vi "上下管柱装配.vi"() -> ()   [LabVIEW 2020]
uses:
  Global_Variable/A131258.vi
  Global_Variable/Global.vi
  Database/Global1.vi
  <vilib>/addons/database/NI_Database_API.lvlib
  <vilib>/addons/database/Connection.llb/Conn Execute.vi
  <vilib>/addons/database/Recordset.llb/Rec Fetch Recordset Data (R).vi
  <vilib>/addons/database/Connection.llb/DB Tools Open Connec (String).vi
panel:
  in  "STEP":string
  out "左压装下限":dbl format="%#.2f"
  out "左压装上限":dbl format="%#.2f"
  out "左下限2":dbl format="%#.2f"
  out "左上限2":dbl format="%#.2f"
  out "左下限1":dbl format="%#.2f"
  out "左上限1":dbl format="%#.2f"
  out "压装最大位移(mm)":dbl
  out "判定结果":bool
  out "位移区间最大压力(KN)":dbl
  out "位移区间最小压力(KN)":dbl
  out "标尺改变":refnum<user-event>
  out "试验项":refnum<user-event>
  out "上序结果":string
  out "RIGHTMIN压力":string
  out "RIGHTMAX压力":string
  out "RIGHT位移":string
  out "LEFTMIN压力":string
  out "LEFTMAX压力":string
  out "LEFT位移":string
  out "RESULT":string
  out "PRODUCTID":string
  out "USERID":string
  out "上管柱码":string
  out "前序deviceID":string
  out "deviceID":string
  out "CODE_ID":string
  in  "判定结果 3":bool[][](array[boolean])=[[TRUE]]
  out "选项卡控件 2":enum32{"左工位压装曲线", "右工位压装曲线 ", "参数查看"}(tab)
  out "左工位曲线":cluster{dbl[], dbl[]}[](graph)
  out "右位移下限":dbl format="%#.2f"
  out "右位移上限":dbl format="%#.2f"
  out "右下限2":dbl format="%#.2f"
  out "右上限2":dbl format="%#.2f"
  out "右下限1":dbl format="%#.2f"
  out "右上限1":dbl format="%#.2f"
  out "压装最大位移(mm) 2":dbl
  out "判定结果 2":bool
  out "右工位曲线":cluster{dbl[], dbl[]}[](graph)
  out "位移区间最大压力(KN) 2":dbl
  out "位移区间最小压力(KN) 2":dbl
  in  "删除":bool
  in  "确定":bool
  in  "添加":bool
  in  "退出":bool
  in  "更新":bool
  in  "产品型号":string(combo)
  in  "选项卡控件 3":enum32{"左工位参数", "右工位参数", "产品管理", "用户管理"}(tab)
  in  "左工位坐标轴参数":string[][](table)=[["mm"], ["mm/s"]]
  in  "左工位判定框参数":string[][](table)=[["mm"], ["mm/s"]]
  in  "左工位结果判定参数":string[][](table)=[["mm"], ["mm/s"]]
  in  "右工位结果判定参数":string[][](table)=[["mm"], ["mm/s"]]
  in  "右工位判定框参数":string[][](table)=[["mm"], ["mm/s"]]
  in  "右工位坐标轴参数":string[][](table)=[["mm"], ["mm/s"]]
  in  "确定按钮":bool
  # "上限"
  # "下限"
  # "上序状态"
  # "上限"
  # "下限"
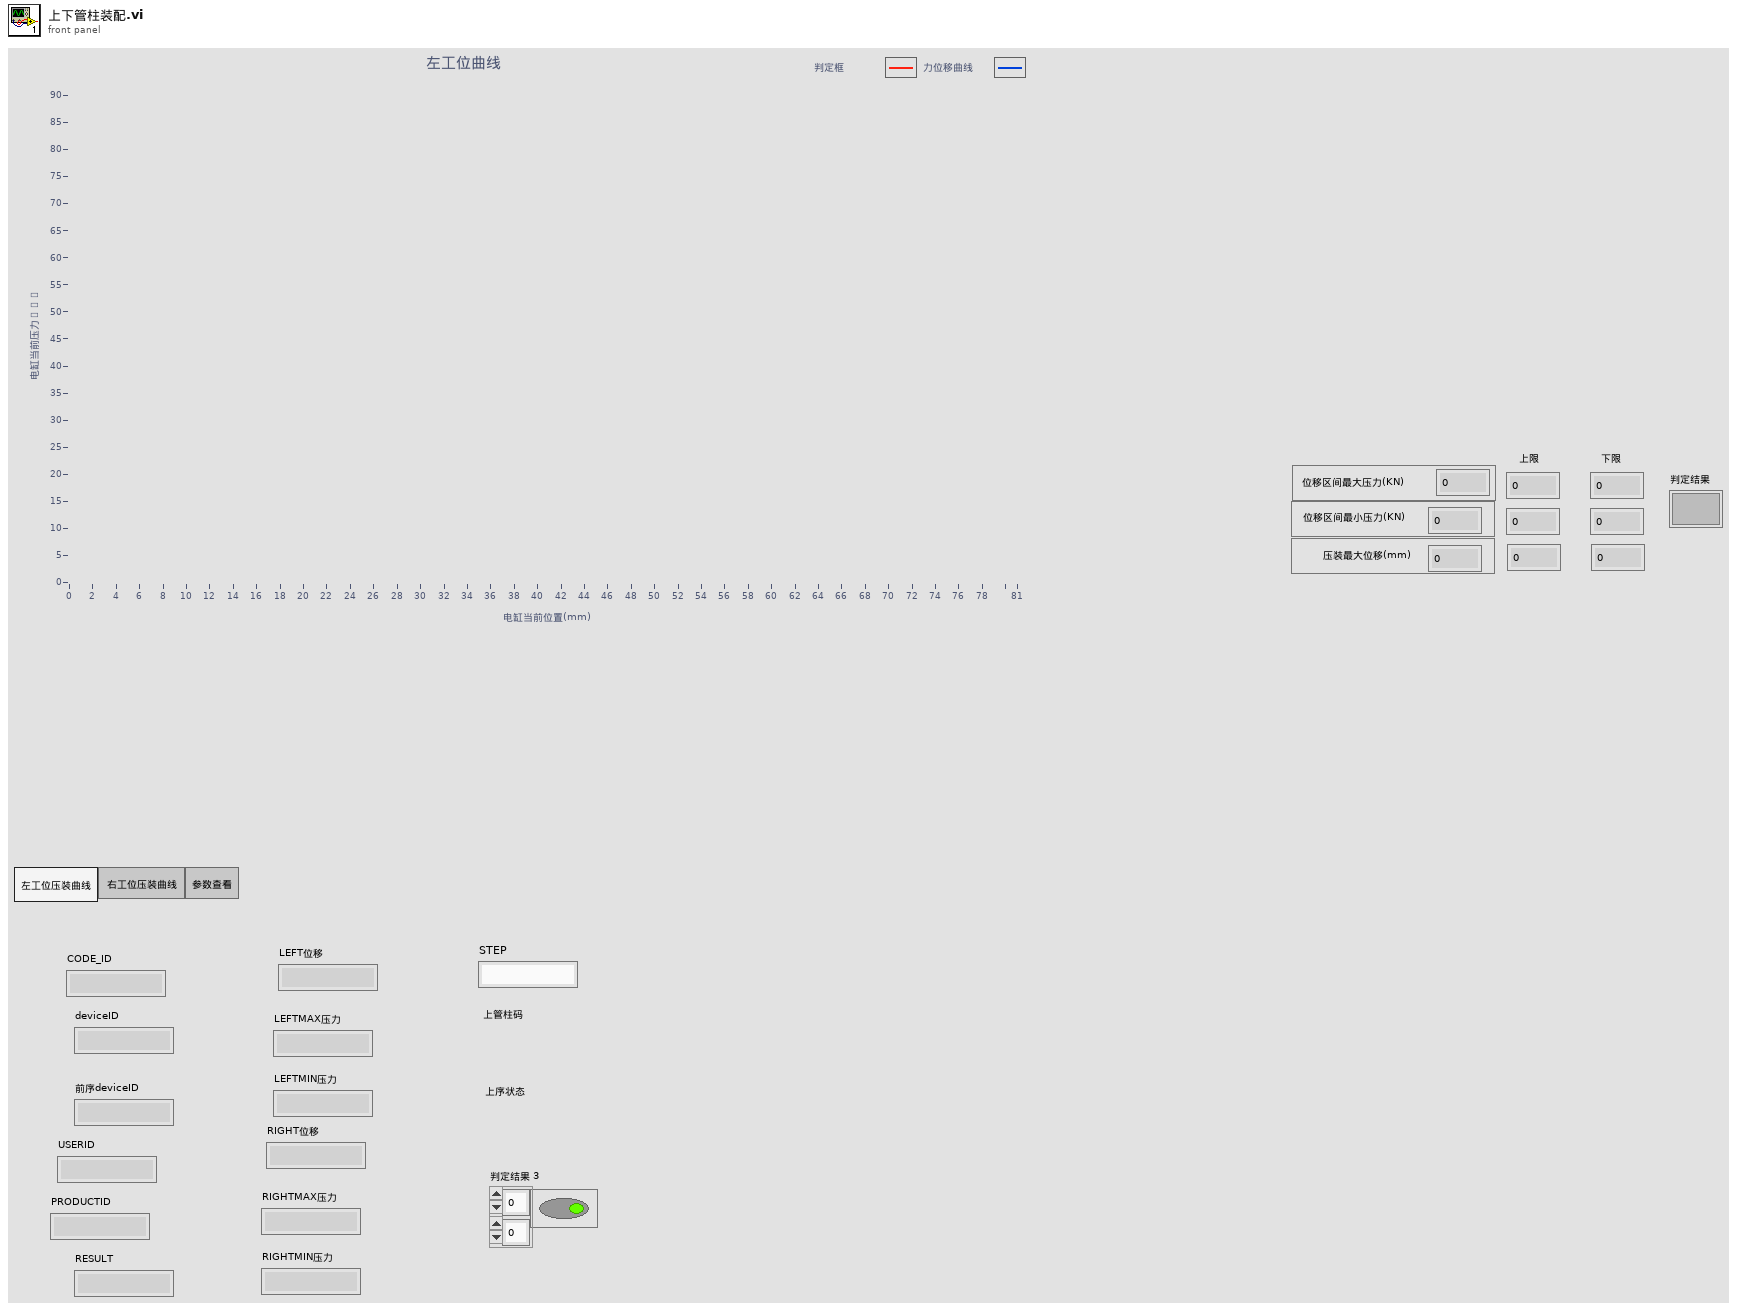
[diagram p1: front panel]
types:
  T1 = cluster{"X ":cluster{"单位":string, "下限":dbl, "上限":dbl}, "Y":cluster{"单位":string, "下限":dbl, "上限":dbl}}
  T2 = cluster{"左工位最大压力 ":cluster{"单位":string, "下限":dbl, "上限":dbl}, "左工位最小压力":cluster{"单位":string, "下限":dbl, "上限":dbl}, "左工位最终压装位移":cluster{"单位":string, "下限":dbl, "上限":dbl}}
  T3 = cluster{"右工位最大压力 ":cluster{"单位":string, "下限":dbl, "上限":dbl}, "右工位最小压力":cluster{"单位":string, "下限":dbl, "上限":dbl}, "右工位最最终位移":cluster{"单位":string, "下限":dbl, "上限":dbl}}
  T4 = cluster{i64, i64, "table":string, "压装最大位移(mm) 2":dbl, "右位移下限":dbl, "右位移上限":dbl, "table":string, "RIGHT位移":string}
  T5 = cluster{i64, i64, "table":string, "位移区间最大压力(KN) 2":dbl, "右下限1":dbl, "右上限1":dbl, "table":string, "RIGHTMAX压力":string}
  T6 = cluster{i64, i64, "table":string, "位移区间最小压力(KN) 2":dbl, "右下限2":dbl, "右上限2":dbl, "table":string, "RIGHTMIN压力":string}
  T7 = cluster{i64, i64, "table":string, "位移区间最小压力(KN) 2":dbl, "右下限2":dbl, "右上限2":dbl, "table":string, "RIGHTMIN压力":string}[]
  T8 = typedef "NI_Database_API.lvlib/Conn ObjectReference.ctl" = refnum<k1>
  T9 = cluster{i64, i64, "位移区间最小压力(KN) 2":dbl, "右下限2":dbl, "右上限2":dbl, "table":string, "RIGHTMIN压力":string}
  T10 = cluster{i64, i64, i64, "RESULT":string, "result string":string}
  T11 = cluster{i64, i64, i64, "RESULT":string, "result string":string}[]
  T12 = typedef "NI_Database_API.lvlib/Rec ObjectReference.ctl" = refnum<k1>
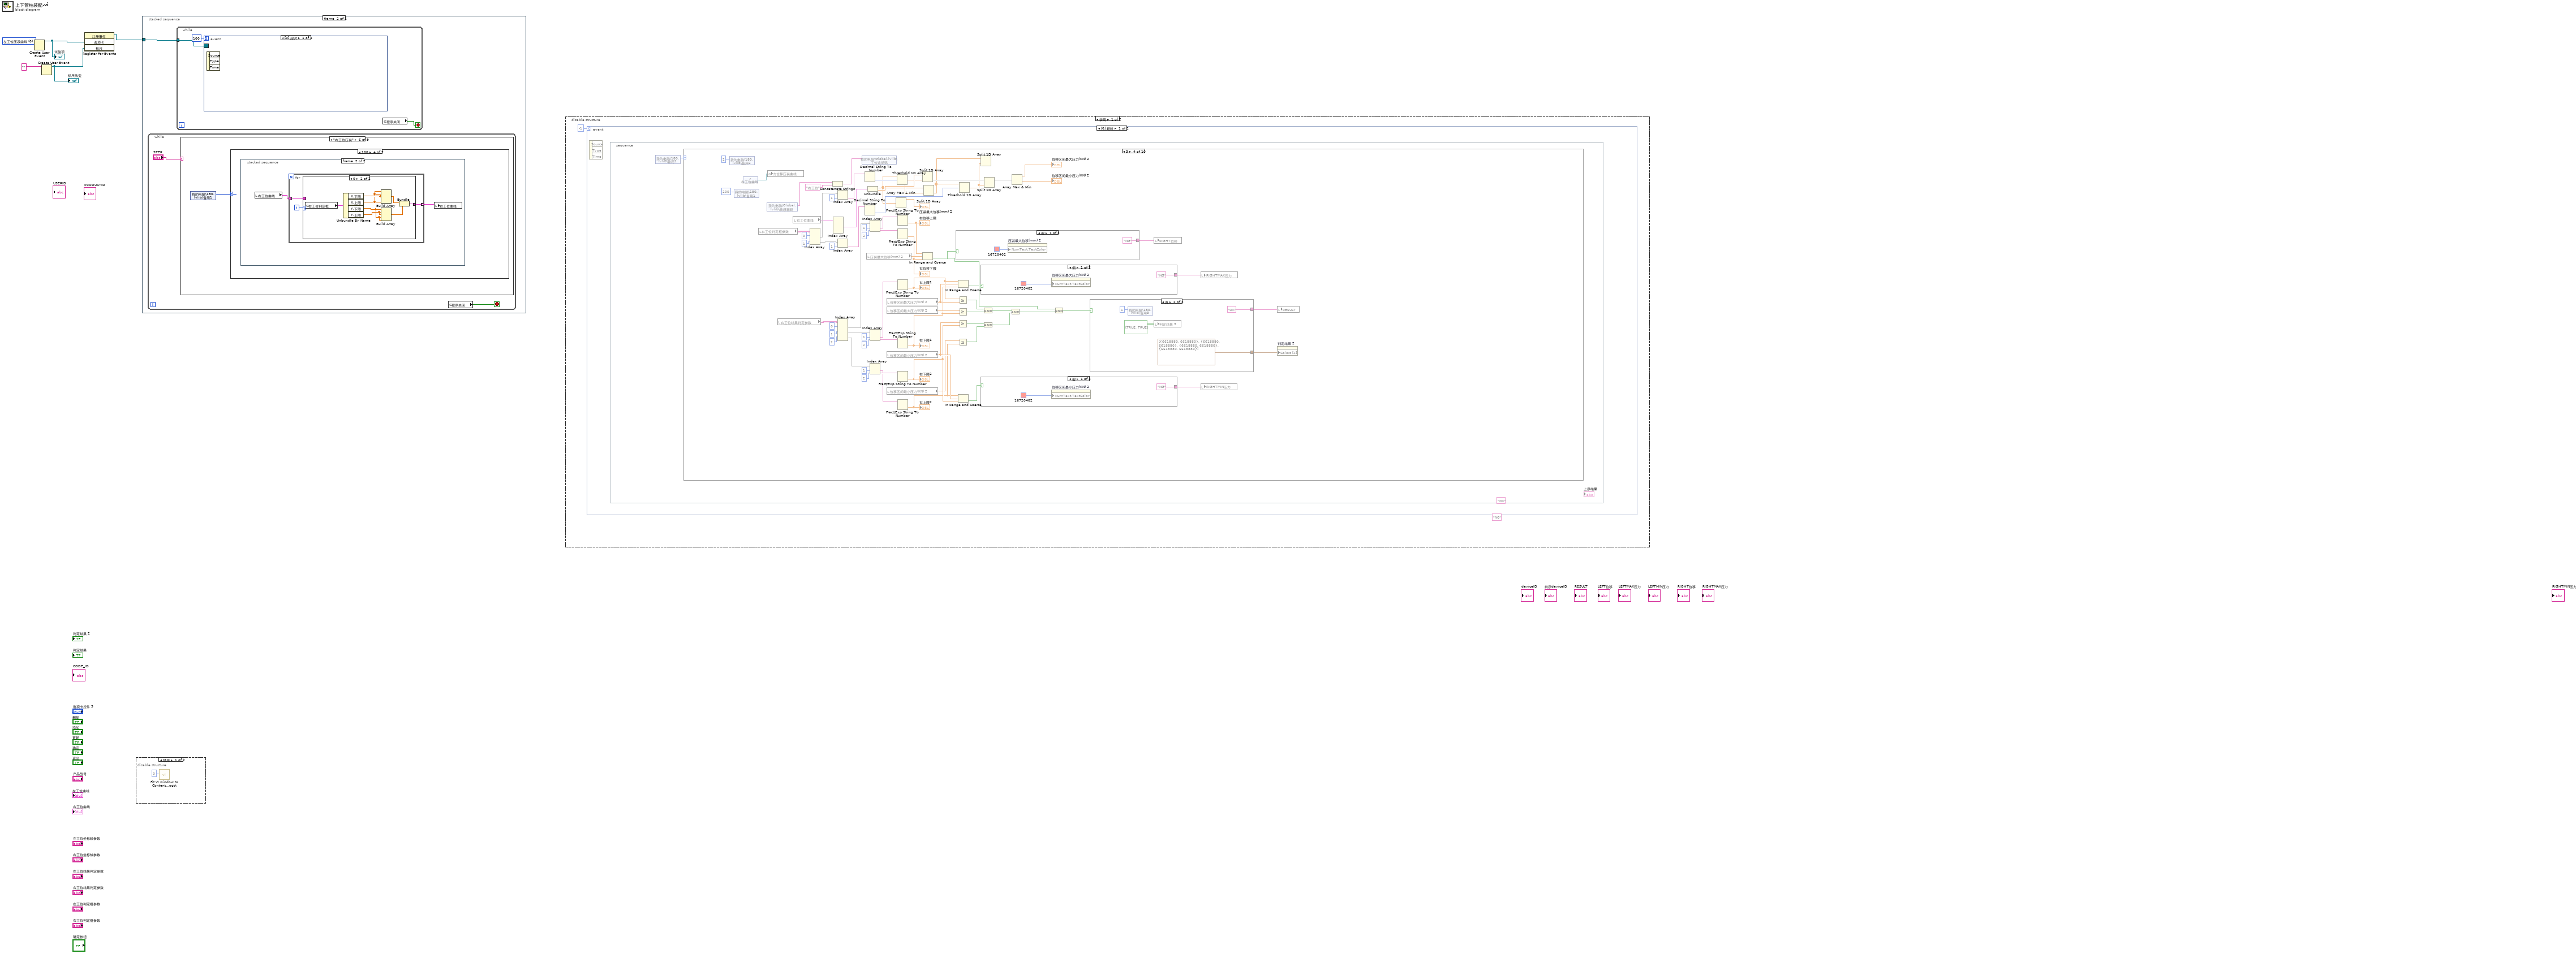
[diagram p0: block diagram]
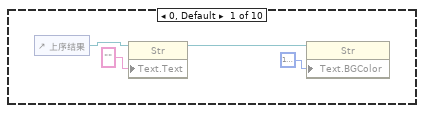
[diagram p2: hidden frame]
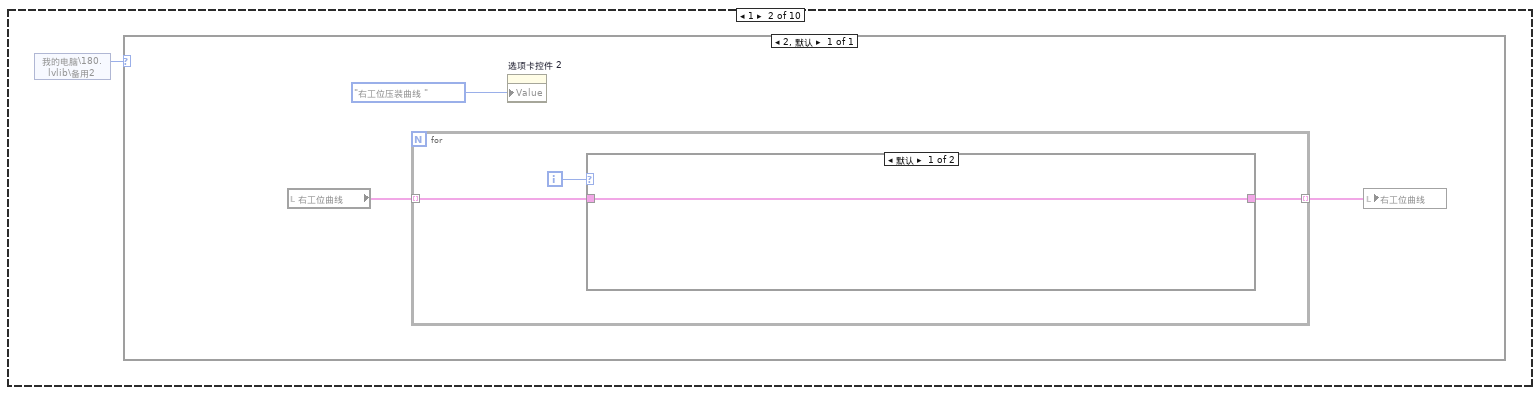
[diagram p3: hidden frame]
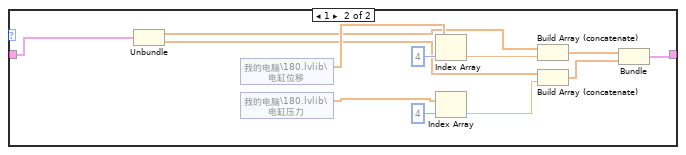
[diagram p4: hidden frame]
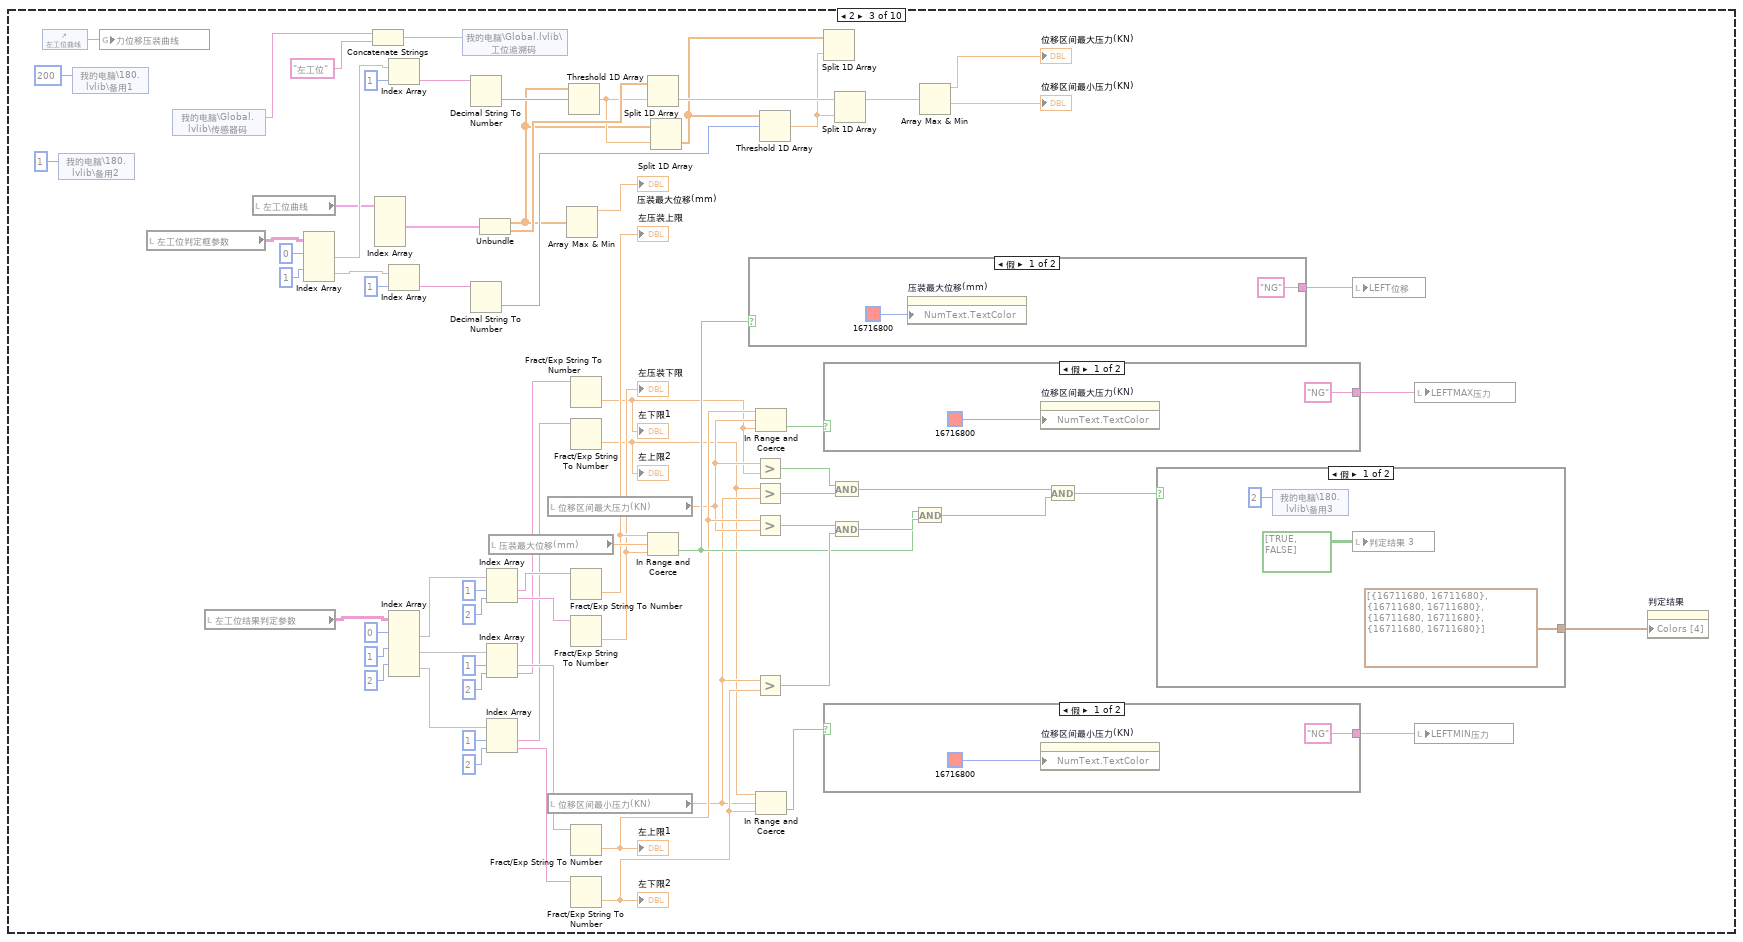
[diagram p5: hidden frame]
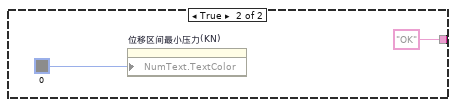
[diagram p6: hidden frame]
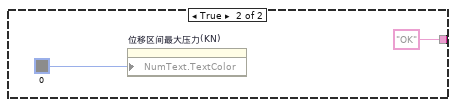
[diagram p7: hidden frame]
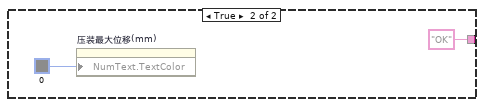
[diagram p8: hidden frame]
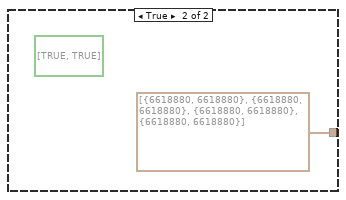
[diagram p9: hidden frame]
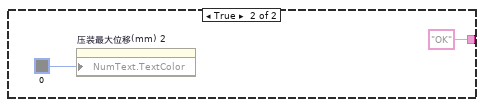
[diagram p10: hidden frame]
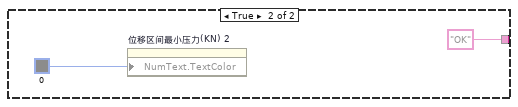
[diagram p11: hidden frame]
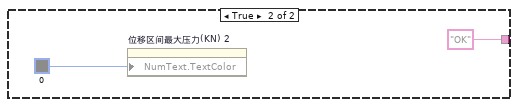
[diagram p12: hidden frame]
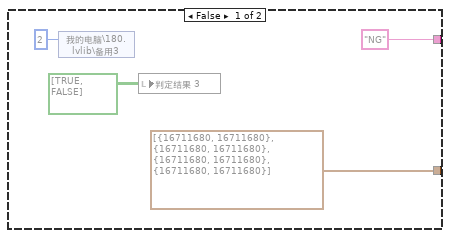
[diagram p13: hidden frame]
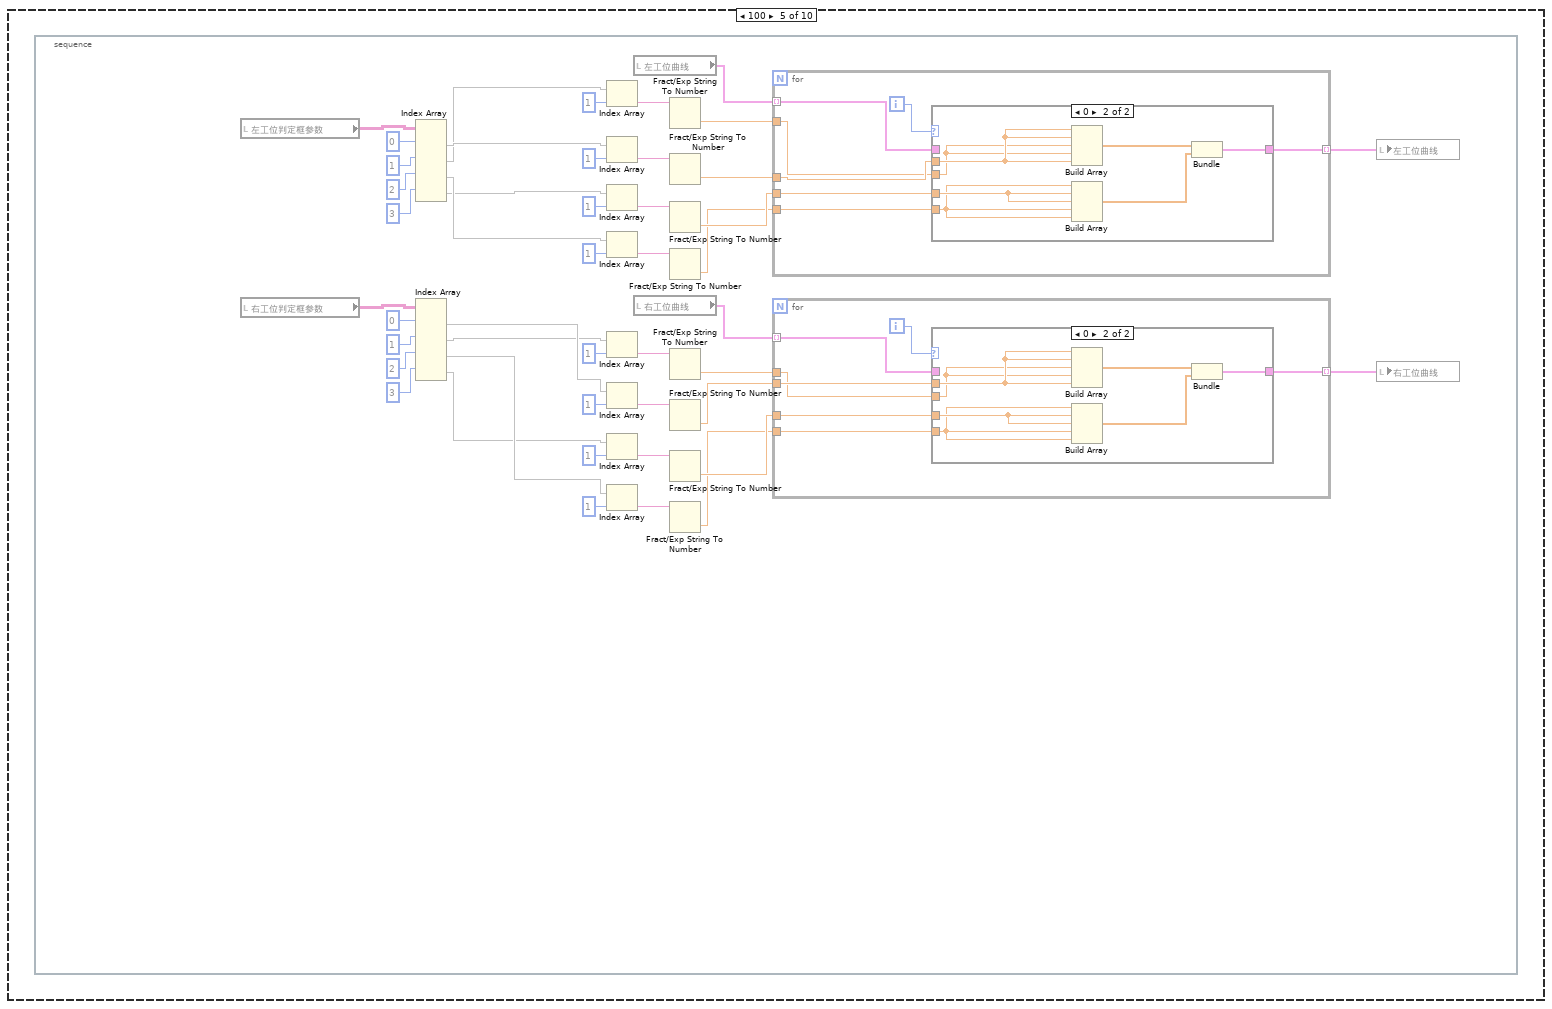
[diagram p14: hidden frame]
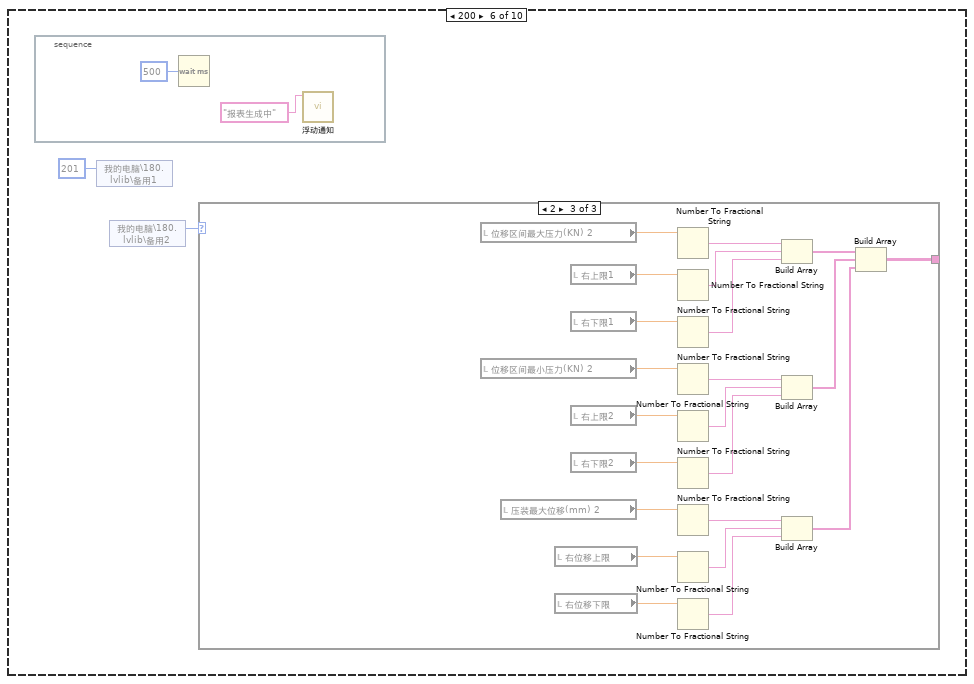
[diagram p17: hidden frame]
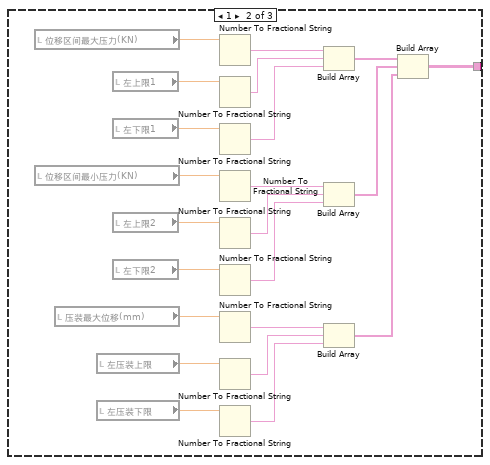
[diagram p19: hidden frame]
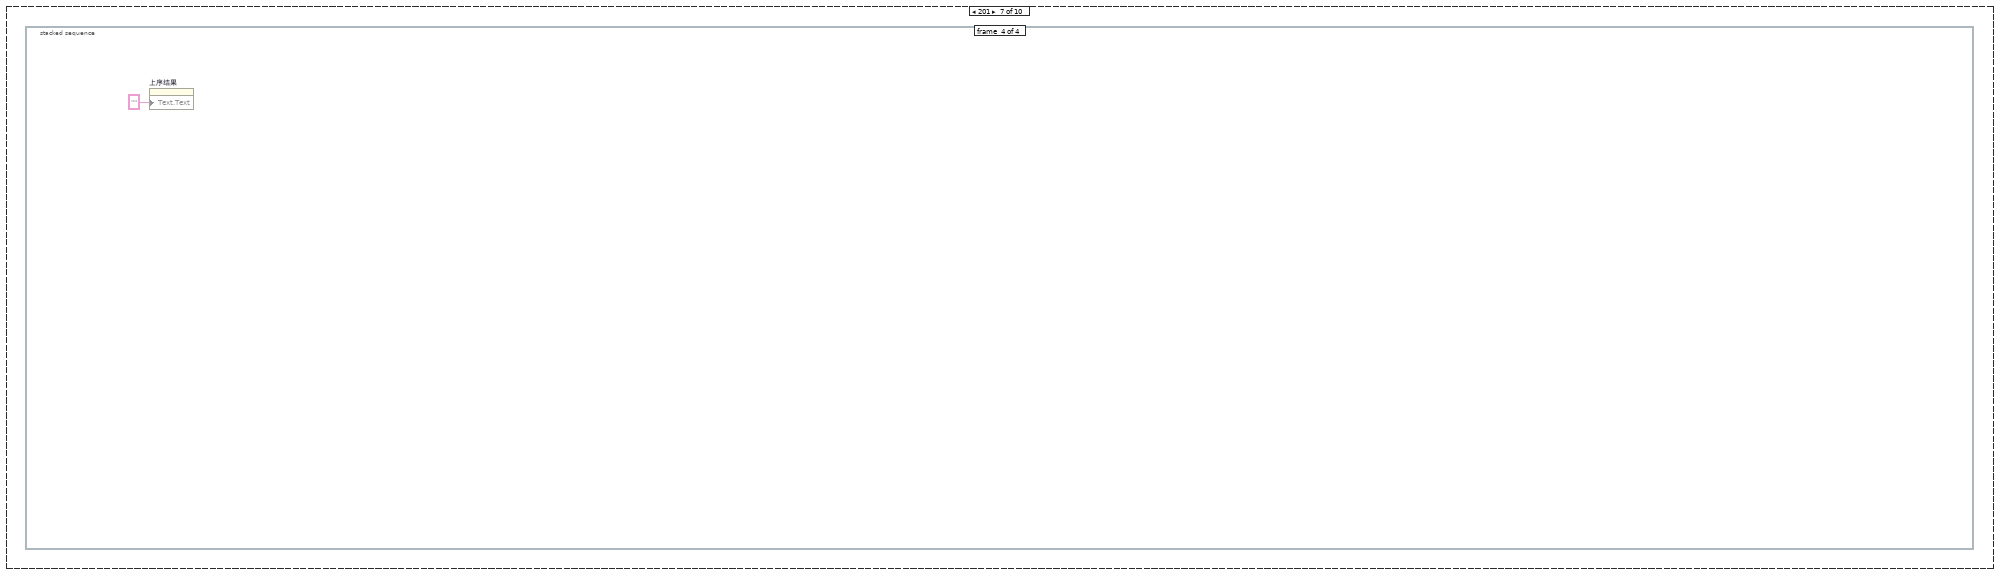
[diagram p20: hidden frame]
diagram:
  w5 = u16 0 items=["左工位压装曲线", "右工位压装曲线", "参数查看"] ("选项卡")
  n1 = Create User Event(user event datatype=w5) -> (user event=w4:refnum<user-event>)  [unwired: 1 in, 1 out]
  "试验项" <- w4
  n2 = Create User Event(user event datatype="" ("标尺")) -> (user event=w1:refnum<user-event>)  [unwired: 1 in, 1 out]
  "标尺改变" <- w1
  n3 = register-events(w4, w1) -> (reference out=w3:refnum<event-registration>)  [unwired: 2 in, 1 out]
  n4 = disable-structure shown="禁用" {
    frame Disabled {
      n5 = call "Fit VI window to Content__ogtk.vi"("border spacing (2 px)"=0) -> ()  [unwired: 5 in, 2 out]
    }
    frame Enabled {
    }
  }
  n6 = stacked-sequence {
    tunnel: w3 -> [_ w12]
    frame #0 {
      n7 = control-ref of="右工位曲线"() -> (w7:refnum<vi>)
      n8 = control-ref of="左工位曲线"() -> (w8:refnum<vi>)
      n9 = for {
        N: 8 -> [_]
        tunnel: [cluster{dbl[], dbl[]} {[], []}] -> w9 mode=indexing
      }
      n10 = global write "A131258.vi" "右工位曲线"(w7) -> ()
      n11 = global write "A131258.vi" "左工位曲线"(w8) -> ()
      n12 = local write "左工位曲线"(w9) -> ()
      n13 = local write "右工位曲线"(w9) -> ()
    }
    frame #1 {
      n14 = while {
        stop <- w28 stop-if-true
        n15 = case shown="\"右工位压装\"" "STEP" {
          frame "等待", Default {
            n16 = local write "STEP"("自动" ("STEP")) -> ()
          }
          frame "自动" {
            n17 = disable-structure shown="禁用" {
              disable-tunnel: [w31 _] -> _
              frame Disabled {
                n18 = global read "Global.vi" "初始化"() -> (w31:bool)
              }
              frame Enabled {
              }
            }
            n19 = shared-variable "我的电脑\\180.lvlib\\备用1"() -> (w30:u16)  [unwired: 1 in, 1 out]
            n20 = case shown="1000" w30 {
              frame 0, Default {
                n21 = call "浮动通知.vi"("通知内容"="等待初始化") -> ()  [unwired: 11 in]
              }
              frame 1000 {
                n22 = local write "STEP"("初始化" ("STEP")) -> ()
                n23 = call "浮动通知.vi"("通知内容"="自动运行中") -> ()  [unwired: 11 in]
              }
            }
          }
          frame "初始化" {
            w40 = -2
            n24 = global read "Global.vi" "Result"() -> (w39:refnum<vi>)
            n25 = Bundle(w40, w40) -> (w38:cluster{i32, i32})  [unwired: 1 in]
            n26 = global write "Global.vi" "当前试验项"(enum16{"左工位", "右工位", "完成"}."左工位" ("当前试验项")) -> ()
            n27 = property class="Tbl"(reference=w39, "Row Headers[]"=string[] [] ("行首字符串[]"), "Value"=string[][] [] ("值"), "Active Cell"=w38, "Cell BG Color"=u32 16777216 ("活动单元格:单元格背景色")) -> ()  [unwired: 1 in, 2 out]
            n28 = local write "STEP"("试验项" ("STEP")) -> ()
            n29 = global read "A131258.vi" "LED-左工位"() -> (w37:refnum<vi>)
            n30 = global read "A131258.vi" "LED-右工位"() -> (w36:refnum<vi>)
            n31 = Wait (ms)(milliseconds to wait=u32 100 ("等待时间（毫秒）")) -> ()  [unwired: 1 out]
            n32 = local write "判定结果 3"(bool[][] [] ("判定结果 3")) -> ()
            n33 = Build Array(w37, w36) -> (w35:refnum<vi>[])
            n34 = for {
              tunnel: w35 -> [w49] mode=indexing
              n35 = property class="Bool"(reference=w49, "Colors [4]"=cluster{u32, u32}[] [{7171459, 7171459}] ("颜色[4]")) -> ()  [unwired: 1 in, 2 out]
            }
          }
          frame "试验项" {
            n36 = global read "Global.vi" "当前试验项"() -> (w51:enum16{"左工位", "右工位", "完成"})
            n37 = case shown="\"左工位\", 默认" w51 {
              selector: w51 -> [w53 _]
              tunnel: [w52 w68] -> w50
              frame "左工位", Default {
                n38 = global read "Global.vi" "试验项目"() -> (w55:bool[])
                n39 = Index Array(array=w55, index=w53) -> (element=w54:bool)
                n40 = case shown="假" w54 {
                  tunnel: [w57 "试验项"] -> w52
                  tunnel: w53 -> [w56 _]
                  frame True {
                    n41 = case shown="\"右工位\"" w56 {
                      tunnel: [w58 w60] -> w57
                      frame "左工位", Default {
                        w58 = "左工位压装"
                        n42 = property on="选项卡控件 2" class="TabCtl (严格)"("Val(Sgnl)"=enum32{"左工位压装曲线", "右工位压装曲线 ", "参数查看"}."左工位压装曲线" ("选项卡控件 2")) -> ()  [unwired: 2 in, 2 out]
                        n43 = call "浮动通知.vi"("通知内容"=w58) -> ()  [unwired: 11 in]
                      }
                      frame "右工位" {
                        w60 = "右工位压装"
                        n44 = property on="选项卡控件 2" class="TabCtl (严格)"("Val(Sgnl)"=enum32{"左工位压装曲线", "右工位压装曲线 ", "参数查看"}."右工位压装曲线 " ("选项卡控件 2")) -> ()  [unwired: 2 in, 2 out]
                        n45 = call "浮动通知.vi"("通知内容"=w60) -> ()  [unwired: 11 in]
                      }
                    }
                  }
                  frame False, Default {
                    n46 = global read "Global.vi" "当前试验项"() -> (w67:enum16{"左工位", "右工位", "完成"})
                    n47 = local read "判定结果 3"() -> (w64:bool[][])
                    n48 = Increment(x=w67) -> (x+1=w66:enum16{"左工位", "右工位", "完成"})
                    n49 = global write "Global.vi" "当前试验项"(w66) -> ()
                    n50 = Build Array (concatenate)(w64, bool[] [FALSE] ("判定结果 3")) -> (w62:bool[][])
                    n51 = local write "判定结果 3"(w62) -> ()
                  }
                }
              }
              frame "完成" {
                w68 = "报表"
                n52 = call "浮动通知.vi"("通知内容"=w68) -> ()  [unwired: 11 in]
              }
            }
            n53 = local write "STEP"(w50) -> ()
          }
          frame "左工位压装" {
            n54 = shared-variable "我的电脑\\180.lvlib\\备用1"() -> (w69:u16)  [unwired: 1 in, 1 out]
            n55 = case shown="1" w69 {
              frame 0, Default {
              }
              frame 1 {
                n56 = shared-variable "我的电脑\\180.lvlib\\备用2"() -> (w70:u16)  [unwired: 1 in, 1 out]
                n57 = case shown="1" w70 {
                  frame 0, Default {
                  }
                  frame 1 {
                    n58 = local read "左工位曲线"() -> (w71:cluster{dbl[], dbl[]}[])
                    n59 = for {
                      tunnel: [w75] -> w72 mode=indexing
                      tunnel: w71 -> [w74] mode=indexing
                      i -> [w73]
                      n60 = case shown="1" w73 {
                        tunnel: [w76 w80] -> w75
                        tunnel: w74 -> [w76 w79]
                        frame Default {
                        }
                        frame 1 {
                          n61 = shared-variable "我的电脑\\180.lvlib\\电缸压力"() -> (w88:sgl[])  [unwired: 1 in, 1 out]
                          n62 = shared-variable "我的电脑\\180.lvlib\\电缸位移"() -> (w86:sgl[])  [unwired: 1 in, 1 out]
                          n63 = Unbundle(w79) -> (w84:dbl[], w83:dbl[])
                          n64 = Index Array(array=w86, index=4) -> (element=w77:sgl)
                          n65 = Index Array(array=w88, index=4) -> (element=w78:sgl)
                          n66 = Build Array (concatenate)(w84, w77) -> (w82:dbl[])
                          n67 = Build Array (concatenate)(w83, w78) -> (w81:dbl[])
                          n68 = Bundle(w82, w81) -> (w80:cluster{dbl[], dbl[]})  [unwired: 1 in]
                        }
                      }
                    }
                    n69 = local write "左工位曲线"(w72) -> ()
                  }
                }
              }
              frame 2 {
                n70 = Wait (ms)(milliseconds to wait=u32 100 ("等待时间（毫秒）")) -> ()  [unwired: 1 out]
                n71 = local write "STEP"("判定" ("STEP")) -> ()
              }
              frame 100 {
                n72 = stacked-sequence {
                  frame #0 {
                    n73 = for {
                      N: 4 -> [_]
                      tunnel: [cluster{dbl[], dbl[]} {[], []}] -> w91 mode=indexing
                    }
                    n74 = local write "左工位曲线"(w91) -> ()
                  }
                  frame #1 {
                    n75 = local read "左工位曲线"() -> (w95:cluster{dbl[], dbl[]}[])
                    n76 = for {
                      tunnel: [w97] -> w94 mode=indexing
                      tunnel: w95 -> [w96] mode=indexing
                      i -> [w98]
                      n77 = case shown="0" w98 {
                        tunnel: [w99 w101] -> w97
                        tunnel: w96 -> [w99 _]
                        frame Default {
                        }
                        frame 0 {
                          n78 = global read "Global.vi" "左工位判定框"() -> (w107:T1)
                          n79 = Unbundle By Name(w107) -> ("X.下限"=w104:dbl, "X.上限"=w100:dbl, "Y.下限"=w105:dbl, "Y.上限"=w106:dbl)
                          n80 = Build Array(w100, w100, w104, w104, w100) -> (w102:dbl[])
                          n81 = Build Array(w105, w106, w106, w105, w105) -> (w103:dbl[])
                          n82 = Bundle(w102, w103) -> (w101:cluster{dbl[], dbl[]})  [unwired: 1 in]
                        }
                      }
                    }
                    n83 = local write "左工位曲线"(w94) -> ()
                  }
                }
              }
              frame 1000 {
                n84 = shared-variable "我的电脑\\180.lvlib\\备用1"(u16 1001 ("备用1")) -> ()  [unwired: 1 in, 1 out]
                n85 = local write "STEP"("扫码" ("STEP")) -> ()
              }
              frame 1002 {
                w116 = -2
                n86 = global read "Global.vi" "Result"() -> (w118:refnum<vi>)
                n87 = Bundle(w116, w116) -> (w117:cluster{i32, i32})  [unwired: 1 in]
                n88 = property class="Tbl"(reference=w118, "Row Headers[]"=string[] [] ("行首字符串[]"), "Value"=string[][] [] ("值"), "Active Cell"=w117, "Cell BG Color"=u32 16777216 ("活动单元格:单元格背景色")) -> ()  [unwired: 1 in, 2 out]
                n89 = global read "A131258.vi" "LED-左工位"() -> (w112:refnum<vi>)
                n90 = global read "A131258.vi" "LED-右工位"() -> (w111:refnum<vi>)
                n91 = Build Array(w112, w111) -> (w110:refnum<vi>[])
                n92 = for {
                  tunnel: w110 -> [w120] mode=indexing
                  n93 = property class="Bool"(reference=w120, "Colors [4]"=cluster{u32, u32}[] [{9868950, 9868950}] ("颜色[4]")) -> ()  [unwired: 1 in, 2 out]
                }
              }
              frame 1001 {
                n94 = global read "Global.vi" "上序状态"() -> (w124:refnum<vi>)
                n95 = shared-variable "我的电脑\\Global.lvlib\\工位追溯码"("" ("工位追溯码")) -> ()  [unwired: 1 in, 1 out]
                n96 = property class="Str"(reference=w124, "Text.Text"="" ("文本.文本"), "Text.BGColor"=u32 16777216 ("文本.文本颜色:背景色")) -> ()  [unwired: 1 in, 2 out]
              }
            }
          }
          frame "右工位压装" {
            n97 = shared-variable "我的电脑\\180.lvlib\\备用1"() -> (w125:u16)  [unwired: 1 in, 1 out]
            n98 = case shown="100" w125 {
              frame 0, Default {
              }
              frame 1 {
                n99 = shared-variable "我的电脑\\180.lvlib\\备用2"() -> (w126:u16)  [unwired: 1 in, 1 out]
                n100 = case shown="2" w126 {
                  frame 0, Default {
                  }
                  frame 2 {
                    n101 = local read "右工位曲线"() -> (w127:cluster{dbl[], dbl[]}[])
                    n102 = for {
                      tunnel: [w131] -> w128 mode=indexing
                      tunnel: w127 -> [w130] mode=indexing
                      i -> [w129]
                      n103 = case shown="1" w129 {
                        tunnel: [w132 w136] -> w131
                        tunnel: w130 -> [w132 w135]
                        frame Default {
                        }
                        frame 1 {
                          n104 = shared-variable "我的电脑\\180.lvlib\\电缸压力"() -> (w144:sgl[])  [unwired: 1 in, 1 out]
                          n105 = shared-variable "我的电脑\\180.lvlib\\电缸位移"() -> (w142:sgl[])  [unwired: 1 in, 1 out]
                          n106 = Unbundle(w135) -> (w140:dbl[], w139:dbl[])
                          n107 = Index Array(array=w142, index=4) -> (element=w133:sgl)
                          n108 = Index Array(array=w144, index=4) -> (element=w134:sgl)
                          n109 = Build Array (concatenate)(w140, w133) -> (w138:dbl[])
                          n110 = Build Array (concatenate)(w139, w134) -> (w137:dbl[])
                          n111 = Bundle(w138, w137) -> (w136:cluster{dbl[], dbl[]})  [unwired: 1 in]
                        }
                      }
                    }
                    n112 = local write "右工位曲线"(w128) -> ()
                  }
                }
              }
              frame 3 {
                w145 = "判定" ("STEP")
                n113 = Wait (ms)(milliseconds to wait=u32 100 ("等待时间（毫秒）")) -> ()  [unwired: 1 out]
                n114 = local write "STEP"(w145) -> ()
                n115 = call "浮动通知.vi"("通知内容"=w145) -> ()  [unwired: 11 in]
              }
              frame 100 {
                n116 = stacked-sequence {
                  frame #0 {
                    n117 = for {
                      N: 4 -> [_]
                      tunnel: [cluster{dbl[], dbl[]} {[], []}] -> w147 mode=indexing
                    }
                    n118 = local write "右工位曲线"(w147) -> ()
                  }
                  frame #1 {
                    n119 = local read "右工位曲线"() -> (w150:cluster{dbl[], dbl[]}[])
                    n120 = for {
                      tunnel: [w153] -> w151 mode=indexing
                      tunnel: w150 -> [w152] mode=indexing
                      i -> [w154]
                      n121 = case shown="0" w154 {
                        tunnel: [w155 w157] -> w153
                        tunnel: w152 -> [w155 _]
                        frame Default {
                        }
                        frame 0 {
                          n122 = global read "Global.vi" "右工位判定框"() -> (w163:T1)
                          n123 = Unbundle By Name(w163) -> ("X.下限"=w160:dbl, "X.上限"=w156:dbl, "Y.下限"=w161:dbl, "Y.上限"=w162:dbl)
                          n124 = Build Array(w156, w156, w160, w160, w156) -> (w158:dbl[])
                          n125 = Build Array(w161, w162, w162, w161, w161) -> (w159:dbl[])
                          n126 = Bundle(w158, w159) -> (w157:cluster{dbl[], dbl[]})  [unwired: 1 in]
                        }
                      }
                    }
                    n127 = local write "右工位曲线"(w151) -> ()
                  }
                }
              }
              frame 1000 {
                n128 = shared-variable "我的电脑\\180.lvlib\\备用1"(u16 1001 ("备用1")) -> ()  [unwired: 1 in, 1 out]
                n129 = local write "STEP"("扫码" ("STEP")) -> ()
              }
              frame 1002 {
                n130 = global read "Global.vi" "试验项目"() -> (w167:bool[])
                n131 = Index Array(array=w167) -> (element=w166:bool)  [unwired: 1 in]
                n132 = case shown="假" w166 {
                  frame False {
                    w172 = -2
                    n133 = global read "Global.vi" "Result"() -> (w171:refnum<vi>)
                    n134 = Bundle(w172, w172) -> (w170:cluster{i32, i32})  [unwired: 1 in]
                    n135 = property class="Tbl"(reference=w171, "Row Headers[]"=string[] [] ("行首字符串[]"), "Value"=string[][] [] ("值"), "Active Cell"=w170, "Cell BG Color"=u32 16777216 ("活动单元格:单元格背景色")) -> ()  [unwired: 1 in, 2 out]
                  }
                  frame True {
                  }
                }
                n136 = global read "A131258.vi" "LED-右工位"() -> (w168:refnum<vi>)
                n137 = property class="Bool"(reference=w168, "Colors [4]"=cluster{u32, u32}[] [{9868950, 9868950}] ("颜色[4]")) -> ()  [unwired: 1 in, 2 out]
              }
              frame 1001 {
                n138 = global read "Global.vi" "上序状态"() -> (w179:refnum<vi>)
                n139 = shared-variable "我的电脑\\Global.lvlib\\工位追溯码"("" ("工位追溯码")) -> ()  [unwired: 1 in, 1 out]
                n140 = property class="Str"(reference=w179, "Text.Text"="" ("文本.文本"), "Text.BGColor"=u32 16777216 ("文本.文本颜色:背景色")) -> ()  [unwired: 1 in, 2 out]
              }
            }
          }
          frame "扫码" {
            n141 = stacked-sequence {
              frame #0 {
                w182 = "请扫管柱码" ("通知内容")
                n142 = global read "Global1.vi" "联机模式"() -> (w180:enum16{"单机", "追溯"})
                n143 = call "浮动通知.vi"("通知内容"=w182) -> ()  [unwired: 11 in]
                n144 = call "输入框.vi"("提示信息"=w182) -> ("条形码输出"=w181:string)
                n145 = case shown="默认" w181 {
                  tunnel: w181 -> [_ w183]
                  tunnel: w180 -> [_ w184]
                  frame "”，“exit" {
                  }
                  frame Default {
                    n146 = case shown="\"追溯\"" w184 {
                      tunnel: [w187 w195] -> w185
                      tunnel: w183 -> [_ w193]
                      frame "单机", Default {
                        n147 = global read "Global.vi" "当前试验项"() -> (w186:enum16{"左工位", "右工位", "完成"})
                        n148 = case shown="\"左工位\", 默认" w186 {
                          tunnel: ["左工位压装" ("文本.文本") "右工位压装" ("文本.文本")] -> w187
                          frame "左工位", Default {
                            n149 = shared-variable "我的电脑\\180.lvlib\\备用1"(u16 1002 ("备用1")) -> ()  [unwired: 1 in, 1 out]
                          }
                          frame "右工位" {
                            n150 = shared-variable "我的电脑\\180.lvlib\\备用1"(u16 1002 ("备用1")) -> ()  [unwired: 1 in, 1 out]
                          }
                        }
                      }
                      frame "追溯" {
                        n151 = global read "Global.vi" "PRODUCT_ID"() -> (w197:string)
                        n152 = call "Get_CODE_ID.vi"("CODE_MAIN"=w193) -> ("CODE_ID"=w192:string)  [unwired: 10 in]
                        n153 = global write "Global.vi" "CODE_ID"(w192) -> ()
                        n154 = call "GET_PRESTATUS.vi"("CODE_ID"=w192, "PRODUCT_ID"=w197) -> ("字符串"=w194:string, "OK?"=w196:bool)  [unwired: 8 in]
                        n155 = case shown="真" w196 {
                          tunnel: [w198 w209] -> w195
                          tunnel: w194 -> [w199 _]
                          frame False {
                            n156 = case shown="\"\", 默认" w199 {
                              tunnel: ["扫码" "扫码"] -> w198
                              frame "", Default {
                                n157 = global read "Global.vi" "上序状态"() -> (w202:refnum<vi>)
                                n158 = property class="Str"(reference=w202, "Text.Text"="漏序" ("文本.文本"), "Text.BGColor"=u32 16776960 ("文本.文本颜色:背景色")) -> ()  [unwired: 1 in, 2 out]
                              }
                              frame "NG" {
                                n159 = global read "Global.vi" "上序状态"() -> (w207:refnum<vi>)
                                n160 = property class="Str"(reference=w207, "Text.Text"="不合格" ("文本.文本"), "Text.BGColor"=u32 16711680 ("文本.文本颜色:背景色")) -> ()  [unwired: 1 in, 2 out]
                              }
                            }
                          }
                          frame True {
                            n161 = global read "Global.vi" "当前试验项"() -> (w208:enum16{"左工位", "右工位", "完成"})
                            n162 = case shown="\"右工位\", 默认" w208 {
                              tunnel: ["右工位压装" ("文本.文本") "左工位压装" ("文本.文本")] -> w209
                              frame "右工位", Default {
                                n163 = global read "Global.vi" "上序状态"() -> (w214:refnum<vi>)
                                n164 = shared-variable "我的电脑\\180.lvlib\\备用1"(u16 1002 ("备用1")) -> ()  [unwired: 1 in, 1 out]
                                n165 = property class="Str"(reference=w214, "Text.Text"="合格" ("文本.文本"), "Text.BGColor"=u32 6618880 ("文本.文本颜色:背景色")) -> ()  [unwired: 1 in, 2 out]
                              }
                              frame "左工位" {
                                n166 = global read "Global.vi" "上序状态"() -> (w219:refnum<vi>)
                                n167 = shared-variable "我的电脑\\180.lvlib\\备用1"(u16 1002 ("备用1")) -> ()  [unwired: 1 in, 1 out]
                                n168 = property class="Str"(reference=w219, "Text.Text"="合格" ("文本.文本"), "Text.BGColor"=u32 6618880 ("文本.文本颜色:背景色")) -> ()  [unwired: 1 in, 2 out]
                              }
                            }
                          }
                        }
                      }
                    }
                    n169 = local write "STEP"(w185) -> ()
                  }
                }
                n170 = shared-variable "我的电脑\\Global.lvlib\\工位追溯码"(w181) -> ()  [unwired: 1 in, 1 out]
              }
              frame #1 {
                n171 = Wait (ms)(milliseconds to wait=u32 100 ("等待时间（毫秒）")) -> ()  [unwired: 1 out]
              }
            }
          }
          frame "判定" {
            n172 = stacked-sequence {
              frame #0 {
                n173 = global read "Global.vi" "当前试验项"() -> (w221:enum16{"左工位", "右工位", "完成"})
                n174 = case shown="\"右工位\"" w221 {
                  frame "左工位" {
                    n175 = global read "Global.vi" "左工位判定参数"() -> (w232:T2)
                    n176 = local read "左工位曲线"() -> (w234:cluster{dbl[], dbl[]}[])
                    n177 = global read "Global.vi" "Result"() -> (w233:refnum<vi>)
                    n178 = call "左工位判定.vi"("Result"=w233, "左工位判定"=w232, "XY曲线"=w234) -> ("大小"=w231:i32, "OK？"=w226:bool)  [unwired: 7 in]
                    n179 = Select(t=cluster{u32, u32}[] [{6618880, 6618880}, {6618880, 6618880}, {6618880, 6618880}, {6618880, 6618880}] ("颜色[4]"), s=w226, f=cluster{u32, u32}[] [{16711680, 16711680}, {16711680, 16711680}, {16711680, 16711680}, {16711680, 16711680}] ("颜色[4]")) -> (s? t:f=w228:cluster{u32, u32}[])
                    n180 = global write "Global.vi" "左判定长度"(w231) -> ()
                    n181 = global read "A131258.vi" "LED-左工位"() -> (w227:refnum<vi>)
                    n182 = case shown="假" w226 {
                      frame False {
                        n183 = global read "Global.vi" "当前试验项"() -> (w236:enum16{"左工位", "右工位", "完成"})
                        n184 = shared-variable "我的电脑\\180.lvlib\\备用3"(u16 2 ("备用1")) -> ()  [unwired: 1 in, 1 out]
                        n185 = Increment(x=w236) -> (x+1=w235:enum16{"左工位", "右工位", "完成"})
                        n186 = global write "Global.vi" "当前试验项"(w235) -> ()
                      }
                      frame True {
                        n187 = shared-variable "我的电脑\\180.lvlib\\备用3"(u16 1 ("备用1")) -> ()  [unwired: 1 in, 1 out]
                      }
                    }
                    n188 = Build Array(TRUE ("元素"), w226) -> (w224:bool[])
                    n189 = local read "判定结果 3"() -> (w223:bool[][])
                    n190 = property class="Bool"(reference=w227, "Colors [4]"=w228) -> ()  [unwired: 1 in, 2 out]
                    n191 = Build Array (concatenate)(w223, w224) -> (w222:bool[][])
                    n192 = local write "判定结果 3"(w222) -> ()
                  }
                  frame "右工位" {
                    n193 = global read "Global.vi" "右工位判定参数"() -> (w249:T3)
                    n194 = local read "右工位曲线"() -> (w251:cluster{dbl[], dbl[]}[])
                    n195 = global read "Global.vi" "Result"() -> (w250:refnum<vi>)
                    n196 = call "右工位判定.vi"("Result"=w250, "右工位判定"=w249, "XY曲线"=w251) -> ("大小"=w248:i32, "OK？"=w243:bool)  [unwired: 7 in]
                    n197 = Select(t=cluster{u32, u32}[] [{6618880, 6618880}, {6618880, 6618880}, {6618880, 6618880}, {6618880, 6618880}] ("颜色[4]"), s=w243, f=cluster{u32, u32}[] [{16711680, 16711680}, {16711680, 16711680}, {16711680, 16711680}, {16711680, 16711680}] ("颜色[4]")) -> (s? t:f=w245:cluster{u32, u32}[])
                    n198 = global write "Global.vi" "右判定长度"(w248) -> ()
                    n199 = global read "A131258.vi" "LED-右工位"() -> (w244:refnum<vi>)
                    n200 = Build Array(TRUE ("元素"), w243) -> (w241:bool[])
                    n201 = local read "判定结果 3"() -> (w240:bool[][])
                    n202 = property class="Bool"(reference=w244, "Colors [4]"=w245) -> ()  [unwired: 1 in, 2 out]
                    n203 = case shown="假" w243 {
                      frame False {
                        n204 = shared-variable "我的电脑\\180.lvlib\\备用3"(u16 2 ("备用1")) -> ()  [unwired: 1 in, 1 out]
                      }
                      frame True {
                        n205 = shared-variable "我的电脑\\180.lvlib\\备用3"(u16 1 ("备用1")) -> ()  [unwired: 1 in, 1 out]
                      }
                    }
                    n206 = Build Array (concatenate)(w240, w241) -> (w239:bool[][])
                    n207 = local write "判定结果 3"(w239) -> ()
                  }
                  frame "完成", Default {
                  }
                }
              }
              frame #1 {
                n208 = global read "Global.vi" "当前试验项"() -> (w256:enum16{"左工位", "右工位", "完成"})
                n209 = Wait (ms)(milliseconds to wait=u32 100 ("等待时间（毫秒）")) -> ()  [unwired: 1 out]
                n210 = local write "STEP"("试验项" ("STEP")) -> ()
                n211 = Increment(x=w256) -> (x+1=w255:enum16{"左工位", "右工位", "完成"})
                n212 = global write "Global.vi" "当前试验项"(w255) -> ()
              }
            }
          }
          frame "报表" {
            n213 = stacked-sequence {
              seq-local: [w258 _ _] -> [_ w270 _]
              frame #0 {
                n214 = shared-variable "我的电脑\\Global.lvlib\\工位追溯码"() -> (w261:string)  [unwired: 1 in, 1 out]
                n215 = call "Report_A131258.vi"("文件重命名"=TRUE, "文件名称"=w261, "布尔数组"="判定结果 3") -> ("工件状态"=w258:string)  [unwired: 7 in, 1 out]
              }
              frame #1 {
                n216 = global read "Global.vi" "Result"() -> (w269:refnum<vi>)
                n217 = property class="Tbl"(reference=w269) -> (reference out=w263:refnum<vi>, "Row Headers[]"=w268:string[])  [unwired: 1 in, 1 out]
                n218 = property class="Tbl"(reference=w263) -> ("Value"=w262:string[][])  [unwired: 1 in, 2 out]
                n219 = for {
                  tunnel: w268 -> [w275] mode=indexing
                  tunnel: w262 -> [w274] mode=indexing
                  tunnel: [w271] -> w267 mode=indexing if=w272
                  n220 = Build Array (concatenate)(w275, w274) -> (w271:string[])
                  n221 = Index Array(array=w274) -> (element=w273:string)  [unwired: 1 in]
                  n222 = case shown="\"\"" w273 {
                    tunnel: [TRUE FALSE] -> w272
                    frame Default {
                    }
                    frame "" {
                    }
                  }
                }
                n223 = global read "Global.vi" "DEVICED_ID"() -> (w265:string)
                n224 = global read "Global.vi" "USER_ID"() -> (w266:string)
                n225 = global read "Global.vi" "CODE_ID"() -> (w264:string)
                n226 = call "UPRESULT.vi"("DEVICE_ID"=w265, "USER_ID"=w266, "CODE_ID"=w264, "RESULT_VALUE"=w270) -> ()  [unwired: 11 in, 1 out]
                n227 = call "UPTEST.vi"("Result"=w267, "CODE_ID"=w264, "DEVICE_ID"=w265) -> ()  [unwired: 6 in, 1 out]
              }
              frame #2 {
                n228 = Wait (ms)(milliseconds to wait=u32 100 ("等待时间（毫秒）")) -> ()  [unwired: 1 out]
                n229 = shared-variable "我的电脑\\180.lvlib\\备用1"(u16 0 ("备用1")) -> ()  [unwired: 1 in, 1 out]
                n230 = local write "STEP"("等待" ("STEP")) -> ()
              }
            }
          }
        }
        n231 = global read "Global.vi" "程序关闭"() -> (w28:bool)
      }
      n232 = while {
        tunnel: w12 -> [w14]
        stop <- w15 stop-if-true
        n233 = event shown="[0] 超时" {
          selector: w14 -> [_ _ _ _]
          dyn-events: _ -> [_ _ _ _]
          timeout: 100 -> [_ _ _ _]
          event Timeout {
            n234 = event-data() -> ()  [unwired: 1 in, 3 out]
          }
          event User Event {
            n235 = event-data() -> ("选项卡"=→"选项卡控件 2":u16)  [unwired: 1 in, 4 out]
          }
          event "左工位曲线", "右工位曲线": Scale Range Change {
            n236 = event-data() -> ("CtlRef"=w19:refnum<vi>)  [unwired: 1 in, 7 out]
            n237 = shared-variable "我的电脑\\Global.lvlib\\产品型号"() -> (w17:string)  [unwired: 1 in, 1 out]
            n238 = call "XY_conf.vi"("方式"=enum16{"写入", "读取"}."写入", "产品"=w17, "XY图引用"=w19) -> ()  [unwired: 4 in, 1 out]
          }
          event User Event {
            n239 = event-data() -> ("标尺"=w23:string)  [unwired: 1 in, 4 out]
            n240 = control-ref of="左工位曲线"() -> (w22:refnum<vi>)
            n241 = control-ref of="右工位曲线"() -> (w21:refnum<vi>)
            n242 = Build Array(w22, w21) -> (w20:refnum<vi>[])
            n243 = for {
              tunnel: w23 -> [w25]
              tunnel: w20 -> [w24] mode=indexing
              n244 = call "XY_conf.vi"("方式"=enum16{"写入", "读取"}."读取", "产品"=w25, "XY图引用"=w24) -> ()  [unwired: 4 in, 1 out]
            }
          }
        }
        n245 = global read "Global.vi" "程序关闭"() -> (w15:bool)
      }
    }
  }
  n246 = disable-structure shown="禁用" {
    frame Disabled {
      (unwired) "NG" ("RESULT")
      (unwired) "OK" ("RESULT")
      n247 = event shown="[0] 超时" {
        selector: _ -> [_ _]
        dyn-events: _ -> [_ _]
        timeout: -1 -> [_ _]
        event Timeout {
          n248 = event-data() -> ()  [unwired: 1 in, 3 out]
          n249 = stacked-sequence {
            frame #0 {
              n250 = shared-variable "我的电脑\\180.lvlib\\备用1"() -> (w282:u16)  [unwired: 1 in, 1 out]
              n251 = case shown="3" w282 {
                frame 0, Default {
                  n252 = control-ref of="上序结果"() -> (w286:refnum<vi>)
                  n253 = property class="Str"(reference=w286, "Text.Text"="" ("文本.文本")) -> (reference out=w284:refnum<vi>)  [unwired: 1 in, 1 out]
                  n254 = property class="Str"(reference=w284, "Text.BGColor"=u32 16777216 ("文本.文本颜色:背景色")) -> ()  [unwired: 1 in, 2 out]
                }
                frame 1 {
                  n255 = shared-variable "我的电脑\\180.lvlib\\备用2"() -> (w287:u16)  [unwired: 1 in, 1 out]
                  n256 = case shown="2, 默认" w287 {
                    frame 2, Default {
                      n257 = local read "右工位曲线"() -> (w289:cluster{dbl[], dbl[]}[])
                      n258 = for {
                        tunnel: [w293] -> w290 mode=indexing
                        tunnel: w289 -> [w292] mode=indexing
                        i -> [w291]
                        n259 = case shown="默认" w291 {
                          tunnel: [w294 w298] -> w293
                          tunnel: w292 -> [w294 w297]
                          frame Default {
                          }
                          frame 1 {
                            n260 = Unbundle(w297) -> (w302:dbl[], w301:dbl[])
                            n261 = shared-variable "我的电脑\\180.lvlib\\电缸位移"() -> (w304:sgl[])  [unwired: 1 in, 1 out]
                            n262 = shared-variable "我的电脑\\180.lvlib\\电缸压力"() -> (w306:sgl[])  [unwired: 1 in, 1 out]
                            n263 = Index Array(array=w304, index=4) -> (element=w295:sgl)
                            n264 = Index Array(array=w306, index=4) -> (element=w296:sgl)
                            n265 = Build Array (concatenate)(w302, w295) -> (w300:dbl[])
                            n266 = Build Array (concatenate)(w301, w296) -> (w299:dbl[])
                            n267 = Bundle(w300, w299) -> (w298:cluster{dbl[], dbl[]})  [unwired: 1 in]
                          }
                        }
                      }
                      n268 = property on="选项卡控件 2" class="TabCtl (严格)"("Value"=enum32{"左工位压装曲线", "右工位压装曲线 ", "参数查看"}."右工位压装曲线 " ("选项卡控件 2")) -> ()  [unwired: 2 in, 2 out]
                      n269 = local write "右工位曲线"(w290) -> ()
                    }
                  }
                }
                frame 2 {
                  n270 = control-ref of="左工位曲线"() -> (w331:refnum<vi>)
                  n271 = shared-variable "我的电脑\\180.lvlib\\备用2"(u16 1 ("备用1")) -> ()  [unwired: 1 in, 1 out]
                  n272 = shared-variable "我的电脑\\180.lvlib\\备用1"(u16 200 ("备用1")) -> ()  [unwired: 1 in, 1 out]
                  n273 = global write "A131258.vi" "力位移压装曲线"(w331) -> ()
                  n274 = local read "左工位判定框参数"() -> (w377:string[][])
                  n275 = shared-variable "我的电脑\\Global.lvlib\\传感器码"() -> (w329:string)  [unwired: 1 in, 1 out]
                  n276 = local read "左工位结果判定参数"() -> (w349:string[][])
                  n277 = local read "左工位曲线"() -> (w372:cluster{dbl[], dbl[]}[])
                  n278 = Index Array(array=w377, index (row) #1=0 ("索引 (行)"), index (row) #2=1 ("索引 (行)")) -> (element #1=w373:string[], element #2=w374:string[])  [unwired: 2 in]
                  n279 = Concatenate Strings(w329, "左工位" ("字符串")) -> (w330:string)
                  n280 = Index Array(array=w372) -> (element #2=w371:cluster{dbl[], dbl[]})  [unwired: 4 in, 3 out]
                  n281 = Index Array(array=w373, index=1 ("索引")) -> (element=w375:string)
                  n282 = Index Array(array=w374, index=1 ("索引")) -> (element=w376:string)
                  n283 = Index Array(array=w349, index (row) #1=0 ("索引 (行)"), index (row) #2=1 ("索引 (行)"), index (row) #3=2 ("索引 (行)")) -> (element #1=w350:string[], element #2=w355:string[], element #3=w319:string[])  [unwired: 3 in]
                  n284 = shared-variable "我的电脑\\Global.lvlib\\工位追溯码"(w330) -> ()  [unwired: 1 in, 1 out]
                  n285 = Decimal String To Number(string=w375) -> (number=w358:i32)  [unwired: 2 in, 1 out]
                  n286 = Decimal String To Number(string=w376) -> (number=w378:i32)  [unwired: 2 in, 1 out]
                  n287 = Unbundle(w371) -> (w356:dbl[], w370:dbl[])
                  n288 = Index Array(array=w350, index #1=1 ("索引"), index #2=2 ("索引")) -> (element #1=w345:string, element #2=w344:string)
                  n289 = Index Array(array=w355, index #1=1 ("索引"), index #2=2 ("索引")) -> (element #1=w343:string, element #2=w342:string)
                  n290 = Index Array(array=w319, index #1=1 ("索引"), index #2=2 ("索引")) -> (element #1=w318:string, element #2=w317:string)
                  n291 = local read "压装最大位移(mm)"() -> (w346:dbl)
                  n292 = local read "位移区间最大压力(KN)"() -> (w315:dbl)
                  n293 = local read "位移区间最小压力(KN)"() -> (w313:dbl)
                  n294 = Array Max & Min(array=w356) -> (max value=→"压装最大位移(mm)":dbl)  [unwired: 3 out]
                  n295 = Threshold 1D Array(2:w358, 3:w356) -> (0:w369:dbl)  [unwired: 1 in]
                  n296 = Fract/Exp String To Number(string=w342) -> (number=w314:dbl)  [unwired: 3 in, 1 out]
                  "左下限1" <- w314
                  n297 = Fract/Exp String To Number(string=w318) -> (number=w312:dbl)  [unwired: 3 in, 1 out]
                  "左上限2" <- w312
                  n298 = Fract/Exp String To Number(string=w345) -> (number=w337:dbl)  [unwired: 3 in, 1 out]
                  "左压装上限" <- w337
                  n299 = Fract/Exp String To Number(string=w344) -> (number=w336:dbl)  [unwired: 3 in, 1 out]
                  "左压装下限" <- w336
                  n300 = Fract/Exp String To Number(string=w343) -> (number=w332:dbl)  [unwired: 3 in, 1 out]
                  "左上限1" <- w332
                  n301 = Fract/Exp String To Number(string=w317) -> (number=w316:dbl)  [unwired: 3 in, 1 out]
                  "左下限2" <- w316
                  n302 = Split 1D Array(array=w370, index=w369) -> (second subarray=w368:dbl[])  [unwired: 1 out]
                  n303 = In Range and Coerce(upper limit=w337, x=w346, lower limit=w336) -> (In Range?=w335:bool)  [unwired: 1 out]
                  n304 = Split 1D Array(array=w356, index=w369) -> (second subarray=w367:dbl[])  [unwired: 1 out]
                  n305 = case shown="假" w335 {
                    tunnel: ["NG" ("RESULT") "OK" ("RESULT")] -> w325
                    frame False {
                      n306 = property on="压装最大位移(mm)" class="DigNum (严格)"("NumText.TextColor"=u32 16716800) -> ()  [unwired: 2 in, 2 out]
                    }
                    frame True {
                      n307 = property on="压装最大位移(mm)" class="DigNum (严格)"("NumText.TextColor"=u32 0) -> ()  [unwired: 2 in, 2 out]
                    }
                  }
                  n308 = Greater?(x=w315, y=w314) -> (0:w311:bool)
                  n309 = Greater?(x=w312, y=w313) -> (0:w310:bool)
                  n310 = Greater?(x=w332, y=w315) -> (0:w341:bool)
                  n311 = Greater?(x=w313, y=w316) -> (0:w340:bool)
                  n312 = In Range and Coerce(upper limit=w332, x=w315, lower limit=w314) -> (In Range?=w334:bool)  [unwired: 1 out]
                  n313 = In Range and Coerce(upper limit=w312, x=w313, lower limit=w316) -> (In Range?=w333:bool)  [unwired: 1 out]
                  n314 = Threshold 1D Array(2:w378, 3:w367) -> (0:w366:dbl)  [unwired: 1 in]
                  n315 = Split 1D Array(array=w367, index=w366) -> ()  [unwired: 2 out]
                  n316 = case shown="假" w334 {
                    tunnel: ["NG" ("RESULT") "OK" ("RESULT")] -> w324
                    frame False {
                      n317 = property on="位移区间最大压力(KN)" class="DigNum (严格)"("NumText.TextColor"=u32 16716800) -> ()  [unwired: 2 in, 2 out]
                    }
                    frame True {
                      n318 = property on="位移区间最大压力(KN)" class="DigNum (严格)"("NumText.TextColor"=u32 0) -> ()  [unwired: 2 in, 2 out]
                    }
                  }
                  n319 = case shown="假" w333 {
                    tunnel: ["NG" ("RESULT") "OK" ("RESULT")] -> w323
                    frame False {
                      n320 = property on="位移区间最小压力(KN)" class="DigNum (严格)"("NumText.TextColor"=u32 16716800) -> ()  [unwired: 2 in, 2 out]
                    }
                    frame True {
                      n321 = property on="位移区间最小压力(KN)" class="DigNum (严格)"("NumText.TextColor"=u32 0) -> ()  [unwired: 2 in, 2 out]
                    }
                  }
                  n322 = And(x=w311, y=w310) -> (x .and. y?=w309:bool)
                  n323 = And(x=w341, y=w340) -> (x .and. y?=w339:bool)
                  n324 = Split 1D Array(array=w368, index=w366) -> (first subarray=w365:dbl[])  [unwired: 1 out]
                  n325 = And(x=w335, y=w339) -> (x .and. y?=w308:bool)
                  n326 = Array Max & Min(array=w365) -> (max value=→"位移区间最大压力(KN)":dbl, min value=→"位移区间最小压力(KN)":dbl)  [unwired: 2 out]
                  n327 = And(x=w309, y=w308) -> (x .and. y?=w307:bool)
                  n328 = case shown="假" w307 {
                    tunnel: [cluster{u32, u32}[] [{16711680, 16711680}, {16711680, 16711680}, {16711680, 16711680}, {16711680, 16711680}] cluster{u32, u32}[] [{6618880, 6618880}, {6618880, 6618880}, {6618880, 6618880}, {6618880, 6618880}]] -> w338
                    frame False {
                      n329 = shared-variable "我的电脑\\180.lvlib\\备用3"(u16 2 ("备用1")) -> ()  [unwired: 1 in, 1 out]
                      n330 = local write "判定结果 3"(bool[][] [[TRUE, FALSE]] ("判定结果")) -> ()
                    }
                    frame True {
                      (unwired) bool[][] [[TRUE, TRUE]] ("判定结果")
                    }
                  }
                  n331 = local write "LEFT位移"(w325) -> ()
                  n332 = local write "LEFTMAX压力"(w324) -> ()
                  n333 = local write "LEFTMIN压力"(w323) -> ()
                  n334 = property on="判定结果" class="Bool (严格)"("Colors [4]"=w338) -> ()  [unwired: 2 in, 2 out]
                }
                frame 3 {
                  n335 = shared-variable "我的电脑\\180.lvlib\\备用2"(u16 2 ("备用1")) -> ()  [unwired: 1 in, 1 out]
                  n336 = shared-variable "我的电脑\\180.lvlib\\备用1"(u16 200 ("备用1")) -> ()  [unwired: 1 in, 1 out]
                  n337 = control-ref of="右工位曲线"() -> (w421:refnum<vi>)
                  n338 = local read "右工位判定框参数"() -> (w455:string[][])
                  n339 = shared-variable "我的电脑\\Global.lvlib\\传感器码"() -> (w419:string)  [unwired: 1 in, 1 out]
                  n340 = global write "A131258.vi" "力位移压装曲线"(w421) -> ()
                  n341 = local read "右工位结果判定参数"() -> (w448:string[][])
                  n342 = local read "右工位曲线"() -> (w456:cluster{dbl[], dbl[]}[])
                  n343 = Index Array(array=w455, index (row) #1=0 ("索引 (行)"), index (row) #2=1 ("索引 (行)")) -> (element #1=w465:string[], element #2=w466:string[])  [unwired: 2 in]
                  n344 = Concatenate Strings(w419, "右工位" ("字符串")) -> (w420:string)
                  n345 = Index Array(array=w456) -> (element #2=w464:cluster{dbl[], dbl[]})  [unwired: 4 in, 3 out]
                  n346 = Index Array(array=w465, index=1 ("索引")) -> (element=w467:string)
                  n347 = Index Array(array=w466, index=1 ("索引")) -> (element=w468:string)
                  n348 = Index Array(array=w448, index (row) #1=0 ("索引 (行)"), index (row) #2=1 ("索引 (行)"), index (row) #3=2 ("索引 (行)")) -> (element #1=w449:string[], element #2=w450:string[], element #3=w408:string[])  [unwired: 3 in]
                  n349 = shared-variable "我的电脑\\Global.lvlib\\工位追溯码"(w420) -> ()  [unwired: 1 in, 1 out]
                  n350 = Decimal String To Number(string=w467) -> (number=w453:i32)  [unwired: 2 in, 1 out]
                  n351 = Decimal String To Number(string=w468) -> (number=w469:i32)  [unwired: 2 in, 1 out]
                  n352 = local read "压装最大位移(mm) 2"() -> (w443:dbl)
                  n353 = Unbundle(w464) -> (w451:dbl[], w463:dbl[])
                  n354 = Index Array(array=w449, index #1=1 ("索引"), index #2=2 ("索引")) -> (element #1=w447:string, element #2=w444:string)
                  n355 = Index Array(array=w450, index #1=1 ("索引"), index #2=2 ("索引")) -> (element #1=w446:string, element #2=w445:string)
                  n356 = Index Array(array=w408, index #1=1 ("索引"), index #2=2 ("索引")) -> (element #1=w406:string, element #2=w407:string)
                  n357 = local read "位移区间最大压力(KN) 2"() -> (w433:dbl)
                  n358 = local read "位移区间最大压力(KN) 2"() -> (w399:dbl)
                  n359 = local read "位移区间最小压力(KN) 2"() -> (w432:dbl)
                  n360 = local read "位移区间最小压力(KN) 2"() -> (w404:dbl)
                  n361 = Array Max & Min(array=w451) -> (max value=→"压装最大位移(mm) 2":dbl)  [unwired: 3 out]
                  n362 = Threshold 1D Array(2:w453, 3:w451) -> (0:w454:dbl)  [unwired: 1 in]
                  n363 = Fract/Exp String To Number(string=w447) -> (number=w439:dbl)  [unwired: 3 in, 1 out]
                  "右位移上限" <- w439
                  n364 = Fract/Exp String To Number(string=w444) -> (number=w438:dbl)  [unwired: 3 in, 1 out]
                  "右位移下限" <- w438
                  n365 = Fract/Exp String To Number(string=w446) -> (number=w434:dbl)  [unwired: 3 in, 1 out]
                  "右上限1" <- w434
                  n366 = Fract/Exp String To Number(string=w445) -> (number=w398:dbl)  [unwired: 3 in, 1 out]
                  "右下限1" <- w398
                  n367 = Fract/Exp String To Number(string=w407) -> (number=w405:dbl)  [unwired: 3 in, 1 out]
                  "右下限2" <- w405
                  n368 = Fract/Exp String To Number(string=w406) -> (number=w403:dbl)  [unwired: 3 in, 1 out]
                  "右上限2" <- w403
                  n369 = Split 1D Array(array=w463, index=w454) -> (second subarray=w462:dbl[])  [unwired: 1 out]
                  n370 = In Range and Coerce(upper limit=w439, x=w443, lower limit=w438) -> (In Range?=w437:bool)  [unwired: 1 out]
                  n371 = Split 1D Array(array=w451, index=w454) -> (second subarray=w461:dbl[])  [unwired: 1 out]
                  n372 = case shown="假" w437 {
                    tunnel: ["NG" ("RESULT") "OK" ("RESULT")] -> w414
                    frame False {
                      n373 = property on="压装最大位移(mm) 2" class="DigNum (严格)"("NumText.TextColor"=u32 16720402) -> ()  [unwired: 2 in, 2 out]
                    }
                    frame True {
                      n374 = property on="压装最大位移(mm) 2" class="DigNum (严格)"("NumText.TextColor"=u32 0) -> ()  [unwired: 2 in, 2 out]
                    }
                  }
                  n375 = Greater Or Equal?(x=w434, y=w433) -> (x >= y?=w396:bool)
                  n376 = Greater Or Equal?(x=w399, y=w398) -> (x >= y?=w395:bool)
                  n377 = Greater Or Equal?(x=w432, y=w405) -> (x >= y?=w401:bool)
                  n378 = Less Or Equal?(x=w404, y=w403) -> (x <= y?=w400:bool)
                  n379 = In Range and Coerce(upper limit=w434, x=w433, lower limit=w398) -> (In Range?=w435:bool)  [unwired: 1 out]
                  n380 = In Range and Coerce(upper limit=w403, x=w432, lower limit=w405) -> (In Range?=w436:bool)  [unwired: 1 out]
                  n381 = Threshold 1D Array(2:w469, 3:w461) -> (0:w460:dbl)  [unwired: 1 in]
                  n382 = Split 1D Array(array=w461, index=w460) -> ()  [unwired: 2 out]
                  n383 = case shown="假" w435 {
                    tunnel: ["NG" ("RESULT") "OK" ("RESULT")] -> w413
                    frame False {
                      n384 = property on="位移区间最大压力(KN) 2" class="DigNum (严格)"("NumText.TextColor"=u32 16720402) -> ()  [unwired: 2 in, 2 out]
                    }
                    frame True {
                      n385 = property on="位移区间最大压力(KN) 2" class="DigNum (严格)"("NumText.TextColor"=u32 0) -> ()  [unwired: 2 in, 2 out]
                    }
                  }
                  n386 = case shown="假" w436 {
                    tunnel: ["NG" ("RESULT") "OK" ("RESULT")] -> w412
                    frame False {
                      n387 = property on="位移区间最小压力(KN) 2" class="DigNum (严格)"("NumText.TextColor"=u32 16720402) -> ()  [unwired: 2 in, 2 out]
                    }
                    frame True {
                      n388 = property on="位移区间最小压力(KN) 2" class="DigNum (严格)"("NumText.TextColor"=u32 0) -> ()  [unwired: 2 in, 2 out]
                    }
                  }
                  n389 = And(x=w396, y=w395) -> (x .and. y?=w397:bool)
                  n390 = And(x=w401, y=w400) -> (x .and. y?=w402:bool)
                  n391 = Split 1D Array(array=w462, index=w460) -> (first subarray=w459:dbl[])  [unwired: 1 out]
                  n392 = And(x=w397, y=w402) -> (x .and. y?=w442:bool)
                  n393 = Array Max & Min(array=w459) -> (max value=→"位移区间最大压力(KN) 2":dbl, min value=→"位移区间最小压力(KN) 2":dbl)  [unwired: 2 out]
                  n394 = And(x=w437, y=w442) -> (x .and. y?=w441:bool)
                  n395 = case shown="真" w441 {
                    tunnel: [cluster{u32, u32}[] [{16711680, 16711680}, {16711680, 16711680}, {16711680, 16711680}, {16711680, 16711680}] cluster{u32, u32}[] [{6618880, 6618880}, {6618880, 6618880}, {6618880, 6618880}, {6618880, 6618880}]] -> w440
                    tunnel: ["NG" ("RESULT") "OK" ("RESULT")] -> w415
                    frame False {
                      n396 = shared-variable "我的电脑\\180.lvlib\\备用3"(u16 2 ("备用1")) -> ()  [unwired: 1 in, 1 out]
                      n397 = local write "判定结果 3"(bool[][] [[TRUE, FALSE]] ("判定结果")) -> ()
                    }
                    frame True {
                      n398 = shared-variable "我的电脑\\180.lvlib\\备用3"(u16 1 ("备用1")) -> ()  [unwired: 1 in, 1 out]
                      n399 = local write "判定结果 3"(bool[][] [[TRUE, TRUE]] ("判定结果")) -> ()
                    }
                  }
                  n400 = local write "RIGHT位移"(w414) -> ()
                  n401 = local write "RIGHTMAX压力"(w413) -> ()
                  n402 = local write "RIGHTMIN压力"(w412) -> ()
                  n403 = local write "RESULT"(w415) -> ()
                  n404 = property on="判定结果 2" class="Bool (严格)"("Colors [4]"=w440) -> ()  [unwired: 2 in, 2 out]
                }
                frame 100 {
                  n405 = stacked-sequence {
                    frame #0 {
                      n406 = local read "左工位判定框参数"() -> (w530:string[][])
                      n407 = local read "右工位判定框参数"() -> (w498:string[][])
                      n408 = Index Array(array=w530, index (row) #1=0 ("索引 (行)"), index (row) #2=1 ("索引 (行)"), index (row) #3=2 ("索引 (行)"), index (row) #4=3 ("索引 (行)")) -> (element #1=w534:string[], element #2=w533:string[], element #3=w532:string[], element #4=w531:string[])  [unwired: 4 in]
                      n409 = Index Array(array=w498, index (row) #1=0 ("索引 (行)"), index (row) #2=1 ("索引 (行)"), index (row) #3=2 ("索引 (行)"), index (row) #4=3 ("索引 (行)")) -> (element #1=w512:string[], element #2=w511:string[], element #3=w510:string[], element #4=w509:string[])  [unwired: 4 in]
                      n410 = Index Array(array=w533, index=1 ("索引")) -> (element=w524:string)
                      n411 = Index Array(array=w534, index=1 ("索引")) -> (element=w525:string)
                      n412 = Index Array(array=w531, index=1 ("索引")) -> (element=w522:string)
                      n413 = Index Array(array=w532, index=1 ("索引")) -> (element=w523:string)
                      n414 = Index Array(array=w511, index=1 ("索引")) -> (element=w503:string)
                      n415 = Index Array(array=w512, index=1 ("索引")) -> (element=w504:string)
                      n416 = Index Array(array=w509, index=1 ("索引")) -> (element=w501:string)
                      n417 = Index Array(array=w510, index=1 ("索引")) -> (element=w502:string)
                      n418 = local read "左工位曲线"() -> (w535:cluster{dbl[], dbl[]}[])
                      n419 = local read "右工位曲线"() -> (w499:cluster{dbl[], dbl[]}[])
                      n420 = Fract/Exp String To Number(string=w524) -> (number=w528:dbl)  [unwired: 3 in, 1 out]
                      n421 = Fract/Exp String To Number(string=w525) -> (number=w529:dbl)  [unwired: 3 in, 1 out]
                      n422 = Fract/Exp String To Number(string=w522) -> (number=w527:dbl)  [unwired: 3 in, 1 out]
                      n423 = Fract/Exp String To Number(string=w523) -> (number=w526:dbl)  [unwired: 3 in, 1 out]
                      n424 = Fract/Exp String To Number(string=w503) -> (number=w507:dbl)  [unwired: 3 in, 1 out]
                      n425 = Fract/Exp String To Number(string=w504) -> (number=w508:dbl)  [unwired: 3 in, 1 out]
                      n426 = Fract/Exp String To Number(string=w501) -> (number=w506:dbl)  [unwired: 3 in, 1 out]
                      n427 = Fract/Exp String To Number(string=w502) -> (number=w505:dbl)  [unwired: 3 in, 1 out]
                      n428 = for {
                        tunnel: [w557] -> w521 mode=indexing
                        tunnel: w535 -> [w556] mode=indexing
                        tunnel: w529 -> [w554]
                        tunnel: w528 -> [w553]
                        tunnel: w527 -> [w552]
                        tunnel: w526 -> [w551]
                        i -> [w555]
                        n429 = case shown="0" w555 {
                          tunnel: [w558 w563] -> w557
                          tunnel: w556 -> [w558 _]
                          tunnel: w554 -> [_ w562]
                          tunnel: w553 -> [_ w561]
                          tunnel: w552 -> [_ w560]
                          tunnel: w551 -> [_ w559]
                          frame Default {
                          }
                          frame 0 {
                            n430 = Build Array(w562, w562, w561, w561, w562) -> (w564:dbl[])
                            n431 = Build Array(w559, w560, w560, w559, w559) -> (w565:dbl[])
                            n432 = Bundle(w564, w565) -> (w563:cluster{dbl[], dbl[]})  [unwired: 1 in]
                          }
                        }
                      }
                      n433 = for {
                        tunnel: [w542] -> w500 mode=indexing
                        tunnel: w499 -> [w541] mode=indexing
                        tunnel: w508 -> [w539]
                        tunnel: w507 -> [w538]
                        tunnel: w506 -> [w537]
                        tunnel: w505 -> [w536]
                        i -> [w540]
                        n434 = case shown="0" w540 {
                          tunnel: [w543 w548] -> w542
                          tunnel: w541 -> [w543 _]
                          tunnel: w539 -> [_ w547]
                          tunnel: w538 -> [_ w546]
                          tunnel: w537 -> [_ w545]
                          tunnel: w536 -> [_ w544]
                          frame Default {
                          }
                          frame 0 {
                            n435 = Build Array(w547, w547, w546, w546, w547) -> (w549:dbl[])
                            n436 = Build Array(w544, w545, w545, w544, w544) -> (w550:dbl[])
                            n437 = Bundle(w549, w550) -> (w548:cluster{dbl[], dbl[]})  [unwired: 1 in]
                          }
                        }
                      }
                      n438 = local write "左工位曲线"(w521) -> ()
                      n439 = local write "右工位曲线"(w500) -> ()
                    }
                  }
                }
                frame 200 {
                  n440 = stacked-sequence {
                    frame #0 {
                      n441 = Wait (ms)(milliseconds to wait=u32 500 ("等待时间（毫秒）")) -> ()  [unwired: 1 out]
                      n442 = call "浮动通知.vi"("通知内容"="报表生成中" ("Status")) -> ()  [unwired: 11 in]
                    }
                  }
                  n443 = shared-variable "我的电脑\\180.lvlib\\备用1"(u16 201 ("备用1")) -> ()  [unwired: 1 in, 1 out]
                  n444 = shared-variable "我的电脑\\180.lvlib\\备用2"() -> (w567:u16)  [unwired: 1 in, 1 out]
                  n445 = case shown="2" w567 {
                    tunnel: [_ w568 w599] -> _
                    frame 0, Default {
                    }
                    frame 1 {
                      n446 = local read "位移区间最大压力(KN)"() -> (w580:dbl)
                      n447 = local read "位移区间最小压力(KN)"() -> (w575:dbl)
                      n448 = local read "压装最大位移(mm)"() -> (w579:dbl)
                      n449 = local read "左压装上限"() -> (w572:dbl)
                      n450 = local read "左压装下限"() -> (w571:dbl)
                      n451 = local read "左上限1"() -> (w577:dbl)
                      n452 = local read "左下限1"() -> (w576:dbl)
                      n453 = local read "左上限2"() -> (w574:dbl)
                      n454 = local read "左下限2"() -> (w573:dbl)
                      n455 = Number To Fractional String(number=w580) -> (F-format string=w589:string)  [unwired: 3 in]
                      n456 = Number To Fractional String(number=w577) -> (F-format string=w588:string)  [unwired: 3 in]
                      n457 = Number To Fractional String(number=w576) -> (F-format string=w583:string)  [unwired: 3 in]
                      n458 = Number To Fractional String(number=w575) -> (F-format string=w586:string)  [unwired: 3 in]
                      n459 = Number To Fractional String(number=w574) -> (F-format string=w585:string)  [unwired: 3 in]
                      n460 = Number To Fractional String(number=w573) -> (F-format string=w582:string)  [unwired: 3 in]
                      n461 = Number To Fractional String(number=w579) -> (F-format string=w578:string)  [unwired: 3 in]
                      n462 = Number To Fractional String(number=w572) -> (F-format string=w570:string)  [unwired: 3 in]
                      n463 = Number To Fractional String(number=w571) -> (F-format string=w569:string)  [unwired: 3 in]
                      n464 = Build Array(w589, w588, w583) -> (w587:string[])
                      n465 = Build Array(w586, w585, w582) -> (w584:string[])
                      n466 = Build Array(w578, w570, w569) -> (w581:string[])
                      n467 = Build Array(w587, w584, w581) -> (w568:string[][])
                    }
                    frame 2 {
                      n468 = local read "位移区间最大压力(KN) 2"() -> (w598:dbl)
                      n469 = local read "位移区间最小压力(KN) 2"() -> (w595:dbl)
                      n470 = local read "压装最大位移(mm) 2"() -> (w592:dbl)
                      n471 = local read "右位移上限"() -> (w591:dbl)
                      n472 = local read "右位移下限"() -> (w590:dbl)
                      n473 = local read "右上限1"() -> (w597:dbl)
                      n474 = local read "右下限1"() -> (w596:dbl)
                      n475 = local read "右上限2"() -> (w594:dbl)
                      n476 = local read "右下限2"() -> (w593:dbl)
                      n477 = Number To Fractional String(number=w598) -> (F-format string=w611:string)  [unwired: 3 in]
                      n478 = Number To Fractional String(number=w597) -> (F-format string=w610:string)  [unwired: 3 in]
                      n479 = Number To Fractional String(number=w596) -> (F-format string=w605:string)  [unwired: 3 in]
                      n480 = Number To Fractional String(number=w595) -> (F-format string=w608:string)  [unwired: 3 in]
                      n481 = Number To Fractional String(number=w594) -> (F-format string=w607:string)  [unwired: 3 in]
                      n482 = Number To Fractional String(number=w593) -> (F-format string=w604:string)  [unwired: 3 in]
                      n483 = Number To Fractional String(number=w592) -> (F-format string=w602:string)  [unwired: 3 in]
                      n484 = Number To Fractional String(number=w591) -> (F-format string=w601:string)  [unwired: 3 in]
                      n485 = Number To Fractional String(number=w590) -> (F-format string=w600:string)  [unwired: 3 in]
                      n486 = Build Array(w611, w610, w605) -> (w609:string[])
                      n487 = Build Array(w608, w607, w604) -> (w606:string[])
                      n488 = Build Array(w602, w601, w600) -> (w603:string[])
                      n489 = Build Array(w609, w606, w603) -> (w599:string[][])
                    }
                  }
                }
                frame 201 {
                  n490 = stacked-sequence {
                    frame #0 {
                      n491 = Wait (ms)(milliseconds to wait=u32 800 ("等待时间（毫秒）")) -> ()  [unwired: 1 out]
                      n492 = shared-variable "我的电脑\\180.lvlib\\备用2"() -> (w614:u16)  [unwired: 1 in, 1 out]
                      n493 = case shown="2" w614 {
                        frame 0, Default {
                        }
                        frame 1 {
                          n494 = shared-variable "我的电脑\\Global.lvlib\\工位追溯码"() -> (w618:string)  [unwired: 1 in, 1 out]
                          n495 = Concatenate Strings(w618, "左" ("字符串")) -> (w616:string)
                          n496 = call "Report_A131258.vi"("文件重命名"=TRUE, "文件名称"=w616) -> ()  [unwired: 8 in, 2 out]
                        }
                        frame 2 {
                          n497 = shared-variable "我的电脑\\Global.lvlib\\工位追溯码"() -> (w623:string)  [unwired: 1 in, 1 out]
                          n498 = Concatenate Strings(w623, "右" ("字符串")) -> (w621:string)
                          n499 = local read "判定结果 3"() -> (w620:bool[][])
                          n500 = call "Report_A131258.vi"("文件重命名"=TRUE, "文件名称"=w621, "布尔数组"=w620) -> ()  [unwired: 7 in, 2 out]
                        }
                      }
                    }
                    frame #1 {
                      n501 = shared-variable "我的电脑\\180.lvlib\\备用2"() -> (w625:u16)  [unwired: 1 in, 1 out]
                      n502 = case shown="2" w625 {
                        frame 0, Default {
                        }
                        frame 2 {
                          n503 = global read "Global1.vi" "联机模式"() -> (w626:enum16{"单机", "追溯"})
                          n504 = case shown="\"追溯\"" w626 {
                            tunnel: w626 -> [_ w627]
                            frame "单机", Default {
                            }
                            frame "追溯" {
                              n505 = local read "CODE_ID"() -> (w650:string)
                              n506 = local read "位移区间最大压力(KN) 2"() -> (w640:dbl)
                              n507 = local read "位移区间最小压力(KN) 2"() -> (w634:dbl)
                              n508 = local read "deviceID"() -> (w653:string)
                              n509 = local read "压装最大位移(mm) 2"() -> (w637:dbl)
                              n510 = local read "RIGHTMAX压力"() -> (w630:string)
                              n511 = local read "RIGHTMIN压力"() -> (w631:string)
                              n512 = local read "RIGHT位移"() -> (w629:string)
                              n513 = local read "右位移下限"() -> (w636:dbl)
                              n514 = local read "右位移上限"() -> (w635:dbl)
                              n515 = local read "右下限1"() -> (w639:dbl)
                              n516 = local read "右上限1"() -> (w638:dbl)
                              n517 = local read "右下限2"() -> (w633:dbl)
                              n518 = local read "右上限2"() -> (w632:dbl)
                              n519 = Decimal String To Number(string=w653, default (0L)=i64 0 ("长度")) -> (number=w648:i64)  [unwired: 1 in, 1 out]
                              n520 = Decimal String To Number(string=w650, default (0L)=i64 0 ("长度")) -> (number=w647:i64)  [unwired: 1 in, 1 out]
                              n521 = Bundle(w648, w647, "table"="最大位移", "压装最大位移(mm) 2"=w637, "右位移下限"=w636, "右位移上限"=w635, "table"="mm", "RIGHT位移"=w629) -> (w655:T4)  [unwired: 1 in]
                              n522 = Bundle(w648, w647, "table"="最大压力", "位移区间最大压力(KN) 2"=w640, "右下限1"=w639, "右上限1"=w638, "table"="KN", "RIGHTMAX压力"=w630) -> (w654:T5)  [unwired: 1 in]
                              n523 = Bundle(w648, w647, "table"="最小压力", "位移区间最小压力(KN) 2"=w634, "右下限2"=w633, "右上限2"=w632, "table"="KN", "RIGHTMIN压力"=w631) -> (w628:T6)  [unwired: 1 in]
                              n524 = call "GetSQLstring.vi"("联机模式"=w627) -> ("错误输出"=w657:errorcluster, "连接字符串"=w658:string)  [unwired: 9 in]
                              n525 = Build Array(w655, w654, w628) -> (w649:T7)
                              n526 = call-poly <vilib>:"DB Tools Open Connection.vi"("error in (no error)"=w657, "connection information"=w658) -> ("error out"=w659:errorcluster, "connection reference"=w656:T8)  [unwired: 6 in]
                              n527 = for {
                                tunnel: w649 -> [w664] mode=indexing
                                tunnel: w656 -> [w662]
                                shift-right: [w660] -> _
                                shift-left: w659 -> [w667]
                                w663 = string[] ["DEVICE_ID", "CODE_ID", "TEST_NAME", "TEST_VALUE", "TEST_VALUE_MIN", "TEST_VALUE_MAX", "TEST_VALUE_UNIT", "TEST_VALUE_RESULT"] ("columns")
                                w665 = "Test" ("table")
                                n528 = call <vilib>:"DB Tools Insert Data.vi"("data"=w664, "error in (no error)"=w667, "columns"=w663, "table"=w665, "connection reference"=w662) -> ("error out"=w666:errorcluster, "connection reference out"=w661:T8)  [unwired: 5 in]
                                n529 = case shown="错误" w666 {
                                selector: w666 -> [w668 w694]
                                tunnel: w663 -> [_ w691]
                                tunnel: w661 -> [w669 w676]
                                tunnel: w665 -> [_ w695]
                                tunnel: w664 -> [_ w685]
                                tunnel: [w669 w675] -> _
                                tunnel: [w668 w674] -> w660
                                frame No Error {
                                }
                                frame Error {
                                n530 = Delete From Array(array=w691, length=1 ("长度"), index=2 ("索引")) -> (array with subset deleted=w692:string[])  [unwired: 1 out]
                                n531 = Unbundle(w685) -> (w684:i64, w672:i64, "table"=w677:string, "位移区间最小压力(KN) 2"=w683:dbl, "右下限2"=w682:dbl, "右上限2"=w681:dbl, "table"=w680:string, "RIGHTMIN压力"=w679:string)
                                n532 = Bundle(w684, w672, "位移区间最小压力(KN) 2"=w683, "右下限2"=w682, "右上限2"=w681, "table"=w680, "RIGHTMIN压力"=w679) -> (w678:T9)  [unwired: 1 in]
                                n533 = Number To Decimal String(number=w672) -> (decimal integer string=w671:string)  [unwired: 1 in]
                                n534 = call <vilib>:"Clear Errors.vi"("error in (no error)"=w694) -> ("error out"=w693:errorcluster)  [unwired: 5 in, 1 out]
                                n535 = Concatenate Strings("WHERE ( TEST_NAME ='" ("condition"), w677, "' ", "AND CODE_ID =" ("condition"), w671, ")" ("condition")) -> (w687:string)
                                n536 = call <vilib>:"DB Tools Update Data.vi"("condition"=w687, "data"=w678, "error in (no error)"=w693, "columns"=w692, "table"=w695, "connection reference"=w676) -> ("error out"=w674:errorcluster, "connection reference out"=w675:T8)  [unwired: 4 in]
                                }
                                }
                              }
                            }
                          }
                        }
                      }
                    }
                    frame #2 {
                      n537 = shared-variable "我的电脑\\180.lvlib\\备用2"() -> (w696:u16)  [unwired: 1 in, 1 out]
                      n538 = case shown="2" w696 {
                        frame 0, Default {
                        }
                        frame 2 {
                          n539 = global read "Global1.vi" "联机模式"() -> (w697:enum16{"单机", "追溯"})
                          n540 = case shown="\"追溯\"" w697 {
                            tunnel: w697 -> [_ w698]
                            frame "单机", Default {
                            }
                            frame "追溯" {
                              n541 = Get Date/Time String(date format (0)=enum16{"short", "long", "abbreviated"}."short" ("日期格式(0)"), want seconds? (F)=FALSE ("需要秒？(F)")) -> (date string=w720:string, time string=w721:string)  [unwired: 1 in]
                              n542 = Concatenate Strings(w720, " " ("字符串"), w721) -> (w723:string)
                              n543 = local read "CODE_ID"() -> (w718:string)
                              n544 = local read "deviceID"() -> (w716:string)
                              n545 = local read "USERID"() -> (w724:string)
                              n546 = Search and Replace String(replace all?=TRUE ("替换全部？(F)"), input string=w723, search string="/" ("替换字符串(\"\")"), replace string="-" ("替换字符串(\"\")")) -> (result string=w722:string)  [unwired: 4 in, 3 out]
                              n547 = local read "RESULT"() -> (w699:string)
                              n548 = Decimal String To Number(string=w716, default (0L)=i64 0 ("默认(0 I32)")) -> (number=w717:i64)  [unwired: 1 in, 1 out]
                              n549 = Decimal String To Number(string=w724, default (0L)=i64 0 ("默认(0 I32)")) -> (number=w725:i64)  [unwired: 1 in, 1 out]
                              n550 = Decimal String To Number(string=w718, default (0L)=i64 0 ("默认(0 I32)")) -> (number=w719:i64)  [unwired: 1 in, 1 out]
                              n551 = Bundle(w717, w725, w719, "RESULT"=w699, "result string"=w722) -> (w714:T10)  [unwired: 1 in]
                              n552 = call "GetSQLstring.vi"("联机模式"=w698) -> ("错误输出"=w711:errorcluster, "连接字符串"=w710:string)  [unwired: 9 in]
                              n553 = Build Array(w714) -> (w715:T11)
                              n554 = call-poly <vilib>:"DB Tools Open Connection.vi"("error in (no error)"=w711, "connection information"=w710) -> ("error out"=w709:errorcluster, "connection reference"=w712:T8)  [unwired: 6 in]
                              n555 = for {
                                tunnel: w715 -> [w730] mode=indexing
                                tunnel: w712 -> [w728]
                                shift-right: [w726] -> w713
                                shift-left: w709 -> [w733]
                                w729 = string[] ["DEVICE_ID", "USER_ID", "CODE_ID", "RESULT_VALUE", "RESULT_TIME"] ("columns")
                                w731 = "Result" ("table")
                                n556 = call <vilib>:"DB Tools Insert Data.vi"("data"=w730, "error in (no error)"=w733, "columns"=w729, "table"=w731, "connection reference"=w728) -> ("error out"=w732:errorcluster, "connection reference out"=w727:T8)  [unwired: 5 in]
                                n557 = case shown="错误" w732 {
                                selector: w732 -> [w734 w755]
                                tunnel: w729 -> [_ w752]
                                tunnel: w727 -> [w735 w744]
                                tunnel: w731 -> [_ w756]
                                tunnel: w730 -> [_ w748]
                                tunnel: [w735 w743] -> _
                                tunnel: [w734 w742] -> w726
                                frame No Error {
                                }
                                frame Error {
                                n558 = Array Subset(array=w752, index=3 ("长度"), length=2 ("长度")) -> (w753:string[])
                                n559 = Unbundle(w748) -> (w737:i64, w740:i64, "RESULT"=w747:string, "result string"=w746:string)  [unwired: 1 out]
                                n560 = Number To Decimal String(number=w740) -> (decimal integer string=w741:string)  [unwired: 1 in]
                                n561 = Number To Decimal String(number=w737) -> (decimal integer string=w736:string)  [unwired: 1 in]
                                n562 = Concatenate Strings("WHERE CODE_ID =" ("condition"), w741, "AND DEVICE_ID = ", w736) -> (w749:string)
                                n563 = Bundle("RESULT"=w747, "result string"=w746) -> (w745:cluster{"RESULT":string, "result string":string})  [unwired: 1 in]
                                n564 = call <vilib>:"Clear Errors.vi"("error in (no error)"=w755) -> ("error out"=w754:errorcluster)  [unwired: 5 in, 1 out]
                                n565 = call <vilib>:"DB Tools Update Data.vi"("condition"=w749, "data"=w745, "error in (no error)"=w754, "columns"=w753, "table"=w756, "connection reference"=w744) -> ("error out"=w742:errorcluster, "connection reference out"=w743:T8)  [unwired: 4 in]
                                }
                                }
                              }
                              n566 = call <vilib>:"Simple Error Handler.vi"("error in (no error)"=w713) -> ()  [unwired: 4 in, 5 out]
                            }
                          }
                        }
                      }
                    }
                    frame #3 {
                      n567 = property on="上序结果" class="Str"("Text.Text"="" ("文本.文本")) -> ()  [unwired: 2 in, 2 out]
                    }
                  }
                }
                frame 1000 {
                  n568 = stacked-sequence {
                    frame #0 {
                      (unwired) cluster{u32, u32}[] [{12369084, 12369084}, {12369084, 12369084}, {13816530, 12369084}, {12369084, 13816530}]
                      w761 = "" ("传感器码")
                      n569 = Wait (ms)(milliseconds to wait=u32 300 ("等待时间（毫秒）")) -> ()  [unwired: 1 out]
                      n570 = shared-variable "我的电脑\\180.lvlib\\备用1"(u16 1001 ("备用1")) -> ()  [unwired: 1 in, 1 out]
                      n571 = local write "上管柱码"(w761) -> ()
                      n572 = shared-variable "我的电脑\\Global.lvlib\\传感器码"(w761) -> ()  [unwired: 1 in, 1 out]
                      n573 = property on="上序结果" class="Str"("Text.Text"="" ("字符串")) -> ()  [unwired: 2 in, 2 out]
                    }
                    frame #1 {
                      w763 = "请扫码！" ("通知内容")
                      n574 = call "浮动通知.vi"("通知内容"=w763) -> ()  [unwired: 11 in]
                      n575 = call "输入框.vi"("提示信息"=w763) -> ("条形码输出"=w762:string)
                      "上管柱码" <- w762
                      n576 = shared-variable "我的电脑\\Global.lvlib\\传感器码"(w762) -> ()  [unwired: 1 in, 1 out]
                    }
                  }
                }
                frame 1001 {
                  n577 = global read "Global1.vi" "联机模式"() -> (w764:enum16{"单机", "追溯"})
                  n578 = case shown="\"追溯\"" w764 {
                    frame "单机", Default {
                      n579 = shared-variable "我的电脑\\180.lvlib\\备用1"(u16 1002 ("备用1")) -> ()  [unwired: 1 in, 1 out]
                    }
                    frame "追溯" {
                      n580 = stacked-sequence {
                        frame #0 {
                          w768 = "'" ("字符串")
                          n581 = local read "PRODUCTID"() -> (w767:string)
                          n582 = global read "Global1.vi" "联机模式"() -> (w786:enum16{"单机", "追溯"})
                          n583 = local read "上管柱码"() -> (w770:string)
                          n584 = call "GetSQLstring.vi"("联机模式"=w786) -> ("错误输出"=w784:errorcluster, "连接字符串"=w785:string)  [unwired: 9 in]
                          n585 = Concatenate Strings("SELECT CODE_ID FROM CODE  WHERE CODE_MAIN= '" ("table"), w770, w768, " AND PRODUCT_ID='" ("字符串"), w767, w768) -> (w783:string)
                          n586 = call-poly <vilib>:"DB Tools Open Connection.vi"("error in (no error)"=w784, "connection information"=w785) -> ("error out"=w777:errorcluster, "connection reference"=w778:T8)  [unwired: 6 in]
                          n587 = call-poly <vilib>:"DB Tools Execute Query.vi"("error in (no error)"=w777, "SQL query"=w783, "connection reference"=w778) -> ("error out"=w781:errorcluster, "recordset reference"=w782:T12)  [unwired: 5 in]
                          n588 = call-poly <vilib>:"DB Tools Fetch Recordset Data.vi"("error in (no error)"=w781, "recordset reference"=w782) -> ("error out"=w775:errorcluster, "recordset data"=w780:variant[][])  [unwired: 3 in, 1 out]
                          n589 = Variant To Data(error in=w775, type=string[][] [], Variant=w780) -> (data=w774:string[][])  [unwired: 1 out]
                          n590 = Index Array(array=w774, index (row)=0 ("索引 (行)")) -> (element=w772:string[])  [unwired: 1 in]
                          n591 = Index Array(array=w772, index=0 ("索引 (行)")) -> (element=w766:string)
                          n592 = case shown="\"\"" w766 {
                            frame Default {
                            }
                            frame "" {
                              n593 = control-ref of="上序结果"() -> (w790:refnum<vi>)
                              n594 = property class="Str"(reference=w790, "Text.Text"="漏序" ("字符串")) -> (reference out=w788:refnum<vi>)  [unwired: 1 in, 1 out]
                              n595 = property class="Str"(reference=w788, "Text.BGColor"=u32 16776960 ("文本.文本颜色:背景色")) -> ()  [unwired: 1 in, 2 out]
                            }
                          }
                          n596 = local write "CODE_ID"(w766) -> ()
                        }
                        frame #1 {
                          n597 = global read "Global1.vi" "联机模式"() -> (w812:enum16{"单机", "追溯"})
                          n598 = local read "前序deviceID"() -> (w791:string)
                          n599 = local read "CODE_ID"() -> (w795:string)
                          n600 = call "GetSQLstring.vi"("联机模式"=w812) -> ("错误输出"=w810:errorcluster, "连接字符串"=w811:string)  [unwired: 9 in]
                          n601 = Concatenate Strings("SELECT RESULT_VALUE FROM RESULT  WHERE DEVICE_ID = \n" ("table"), w791, " AND CODE_ID=" ("字符串"), w795) -> (w809:string)
                          n602 = call-poly <vilib>:"DB Tools Open Connection.vi"("error in (no error)"=w810, "connection information"=w811) -> ("error out"=w803:errorcluster, "connection reference"=w804:T8)  [unwired: 6 in]
                          n603 = call-poly <vilib>:"DB Tools Execute Query.vi"("error in (no error)"=w803, "SQL query"=w809, "connection reference"=w804) -> ("error out"=w807:errorcluster, "recordset reference"=w808:T12)  [unwired: 5 in]
                          n604 = call-poly <vilib>:"DB Tools Fetch Recordset Data.vi"("error in (no error)"=w807, "recordset reference"=w808) -> ("error out"=w801:errorcluster, "recordset data"=w806:variant[][])  [unwired: 3 in, 1 out]
                          n605 = Variant To Data(error in=w801, type=string[][] [], Variant=w806) -> (data=w797:string[][], error out=w794:errorcluster)
                          n606 = call <vilib>:"Clear Errors.vi"("error in (no error)"=w794) -> ("error out"=w793:errorcluster)  [unwired: 5 in, 1 out]
                          n607 = Index Array(array=w797, index (row)=0 ("索引 (行)")) -> (element=w799:string[])  [unwired: 1 in]
                          n608 = call <vilib>:"Simple Error Handler.vi"("error in (no error)"=w793) -> ()  [unwired: 4 in, 5 out]
                          n609 = Index Array(array=w799, index=0 ("索引 (行)")) -> (element=w796:string)
                          n610 = case shown="\"NG\"" w796 {
                            frame "假", Default {
                            }
                            frame "OK" {
                              n611 = control-ref of="上序结果"() -> (w816:refnum<vi>)
                              n612 = local read "上管柱码"() -> (w817:string)
                              n613 = property class="Str"(reference=w816, "Text.Text"="合格" ("字符串")) -> (reference out=w814:refnum<vi>)  [unwired: 1 in, 1 out]
                              n614 = String Length(string=w817) -> (length=w820:i32)
                              n615 = Greater?(x=w820, y=4) -> (0:w819:bool)
                              n616 = property class="Str"(reference=w814, "Text.BGColor"=u32 6618880 ("文本.文本颜色:背景色")) -> ()  [unwired: 1 in, 2 out]
                              n617 = case shown="假" w819 {
                                frame False {
                                }
                                frame True {
                                n618 = shared-variable "我的电脑\\180.lvlib\\备用1"(u16 1002 ("备用1")) -> ()  [unwired: 1 in, 1 out]
                                }
                              }
                            }
                            frame "NG" {
                              n619 = control-ref of="上序结果"() -> (w825:refnum<vi>)
                              n620 = property class="Str"(reference=w825, "Text.Text"="不合格" ("字符串")) -> (reference out=w823:refnum<vi>)  [unwired: 1 in, 1 out]
                              n621 = property class="Str"(reference=w823, "Text.BGColor"=u32 16711680 ("文本.文本颜色:背景色")) -> ()  [unwired: 1 in, 2 out]
                            }
                            frame "" {
                              n622 = control-ref of="上序结果"() -> (w829:refnum<vi>)
                              n623 = property class="Str"(reference=w829, "Text.Text"="漏序" ("字符串")) -> (reference out=w828:refnum<vi>)  [unwired: 1 in, 1 out]
                              n624 = property class="Str"(reference=w828, "Text.BGColor"=u32 16776960 ("文本.文本颜色:背景色")) -> ()  [unwired: 1 in, 2 out]
                            }
                          }
                        }
                      }
                    }
                  }
                }
                frame 1002 {
                }
              }
            }
          }
        }
        event Panel Close? {
          n625 = event-data() -> ()  [unwired: 1 in, 4 out]
          n626 = control-ref of="本VI"() -> (w832:refnum<vi>)
          n627 = invoke class="VI" method="FP.Close"(reference=w832) -> (reference out=w830:refnum<vi>, error out=w831:errorcluster)  [unwired: 2 in, 1 out]
          n628 = Close Reference(reference=w830, error in (no error)=w831) -> ()  [unwired: 1 out]
          n629 = event-data("Discard?"=TRUE ("放弃？")) -> ()  [unwired: 1 in, 1 out]
        }
      }
    }
    frame Enabled {
    }
  }
